vi "JTAG Test Panel.vi"() -> ()   [LabVIEW 2010]
uses:
  <vilib>/measure/NI_MABase.lvlib
  <vilib>/Analysis/NI_AALBase.lvlib
panel:
  out "ProgBar":dbl(slide) caption="Send to UUT..." scale=0.0..1.0
  in  "Tab Control":enum32{"General", "Stim"}(tab)=enum."Stim"
  in  "GoStorage":bool
  in  "DCO8MHz":bool
  in  "DCO1Mhz":bool
  in  "InitFirmware":bool
  in  "ResetFirmware":bool
  in  "InitJTAG":bool
  in  "ReadDefaults":bool
  in  "SetDefaults":bool
  out "Power ASIC Trim Values":string[][](table)=[["0x98"], ["0x14"], ["0xFF"], ["0x20"], ["0xFF"], ["0x20"], ["0x2D"], ["0x58"], ["0x1F"], ["0x00"], ["0x77"]]
  in  "BG_CTRL":bool
  in  "CG_CTRL":bool=TRUE
  in  "CG_CTRL 2":u8=170 format="%02x"
  in  "BG_CTRL 2":u8=128 format="%02x"
  in  "BC_CTRL1":u8=28 format="%02x"
  in  "BC_CTRL0":u8=20 max=64 step=1 format="%02x"
  in  "WFD_CTRL":u8=2 format="%02x"
  in  "Pulse Clock":bool
  in  "Pulses":u8=255
  in  "Stop Clock":bool
  in  "Calc Current":bool
  in  "CBAL 26":bool
  in  "UCS/S 26":bool
  in  "Enable 26":bool
  in  "Cal 26":bool
  in  "Current Ch 26":dbl format="%02_4f"
  in  "Direction 26":bool
  in  "Value Ch 26":u16 max=1023 step=1 format="%03x"
  in  "CBAL 25":bool
  in  "UCS/S 25":bool
  in  "Enable 25":bool
  in  "Cal 25":bool
  in  "Current Ch 25":dbl format="%02_4f"
  in  "Direction 25":bool
  in  "Value Ch 25":u16 max=1023 step=1 format="%03x"
  in  "CBAL 24":bool
  in  "UCS/S 24":bool
  in  "Enable 24":bool
  in  "Cal 24":bool
  in  "Current Ch 24":dbl format="%02_4f"
  in  "Direction 24":bool
  in  "Value Ch 24":u16 max=1023 step=1 format="%03x"
  in  "CBAL 23":bool
  in  "UCS/S 23":bool
  in  "Enable 23":bool
  in  "Cal 23":bool
  in  "Current Ch 23":dbl format="%02_4f"
  in  "Direction 23":bool
  in  "Value Ch 23":u16 max=1023 step=1 format="%03x"
  in  "CBAL 22":bool
  in  "UCS/S 22":bool
  in  "Enable 22":bool
  in  "Cal 22":bool
  in  "Current Ch 22":dbl format="%02_4f"
  in  "Direction 22":bool
  in  "Value Ch 22":u16 max=1023 step=1 format="%03x"
  in  "CBAL 21":bool
  in  "UCS/S 21":bool
  in  "Enable 21":bool
  in  "Cal 21":bool
  in  "Current Ch 21":dbl format="%02_4f"
  in  "Direction 21":bool
  in  "Value Ch 21":u16 max=1023 step=1 format="%03x"
  in  "CBAL 20":bool
  in  "UCS/S 20":bool
  in  "Enable 20":bool
  in  "Cal 20":bool
  in  "Current Ch 20":dbl format="%02_4f"
  in  "Direction 20":bool
  in  "Value Ch 20":u16 max=1023 step=1 format="%03x"
  in  "CBAL 19":bool
  in  "UCS/S 19":bool
  in  "Enable 19":bool
  in  "Cal 19":bool
  in  "Current Ch 19":dbl format="%02_4f"
  in  "Direction 19":bool
  in  "Value Ch 19":u16 max=1023 step=1 format="%03x"
  in  "CBAL 18":bool
  in  "UCS/S 18":bool
  in  "Enable 18":bool
  in  "Cal 18":bool
  in  "Current Ch 18":dbl format="%02_4f"
  in  "Direction 18":bool
  in  "Value Ch 18":u16 max=1023 step=1 format="%03x"
  in  "CBAL 17":bool
  in  "UCS/S 17":bool
  in  "Enable 17":bool
  in  "Cal 17":bool
  in  "Current Ch 17":dbl format="%02_4f"
  in  "Direction 17":bool
  in  "Value Ch 17":u16 max=1023 step=1 format="%03x"
  in  "CBAL 16":bool
  in  "UCS/S 16":bool
  in  "Enable 16":bool
  in  "Cal 16":bool
  in  "Current Ch 16":dbl format="%02_4f"
  in  "Direction 16":bool
  in  "Value Ch 16":u16 max=1023 step=1 format="%03x"
  in  "CBAL 15":bool
  in  "UCS/S 15":bool
  in  "Enable 15":bool
  in  "Cal 15":bool
  in  "Current Ch 15":dbl format="%02_4f"
  in  "Direction 15":bool
  in  "Value Ch 15":u16 max=1023 step=1 format="%03x"
  in  "CBAL 14":bool
  in  "UCS/S 14":bool
  in  "Enable 14":bool
  in  "Cal 14":bool
  in  "Current Ch 14":dbl format="%02_4f"
  in  "Direction 14":bool
  in  "Value Ch 14":u16 max=1023 step=1 format="%03x"
  in  "CBAL 13":bool
  in  "UCS/S 13":bool
  in  "Enable 13":bool
  in  "Cal 13":bool
  in  "Current Ch 13":dbl format="%02_4f"
  in  "Direction 13":bool
  in  "Value Ch 13":u16 max=1023 step=1 format="%03x"
  in  "CBAL 12":bool
  in  "UCS/S 12":bool
  in  "Enable 12":bool
  in  "Cal 12":bool
  in  "Current Ch 12":dbl format="%02_4f"
  in  "Direction 12":bool
  in  "Value Ch 12":u16 max=1023 step=1 format="%03x"
  in  "CBAL 11":bool
  in  "UCS/S 11":bool
  in  "Enable 11":bool
  in  "Cal 11":bool
  in  "Current Ch 11":dbl format="%02_4f"
  in  "Direction 11":bool
  in  "Value Ch 11":u16 max=1023 step=1 format="%03x"
  in  "CBAL 10":bool
  in  "UCS/S 10":bool
  in  "Enable 10":bool
  in  "Cal 10":bool
  in  "Current Ch 10":dbl format="%02_4f"
  in  "Direction 10":bool
  in  "Value Ch 10":u16 max=1023 step=1 format="%03x"
  in  "CBAL 9":bool
  in  "UCS/S 9":bool
  in  "Enable 9":bool
  in  "Cal 9":bool
  in  "Current Ch 9":dbl format="%02_4f"
  in  "Direction 9":bool
  in  "Value Ch 9":u16 max=1023 step=1 format="%03x"
  in  "CBAL 8":bool
  in  "UCS/S 8":bool
  in  "Enable 8":bool
  in  "Cal 8":bool
  in  "Current Ch 8":dbl format="%02_4f"
  in  "Direction 8":bool
  in  "Value Ch 8":u16 max=1023 step=1 format="%03x"
  in  "CBAL 7":bool
  in  "UCS/S 7":bool
  in  "Enable 7":bool
  in  "Cal 7":bool
  in  "Current Ch 7":dbl format="%02_4f"
  in  "Direction 7":bool
  in  "Value Ch 7":u16 max=1023 step=1 format="%03x"
  in  "CBAL 6":bool
  in  "UCS/S 6":bool
  in  "Enable 6":bool
  in  "Cal 6":bool
  in  "Current Ch 6":dbl format="%02_4f"
  in  "Direction 6":bool
  in  "Value Ch 6":u16 max=1023 step=1 format="%03x"
  in  "CBAL 5":bool
  in  "UCS/S 5":bool
  in  "Enable 5":bool
  in  "Cal 5":bool
  in  "Current Ch 5":dbl format="%02_4f"
  in  "Direction 5":bool
  in  "Value Ch 5":u16 max=1023 step=1 format="%03x"
  in  "CBAL 4":bool
  in  "UCS/S 4":bool
  in  "Enable 4":bool
  in  "Cal 4":bool
  in  "Current Ch 4":dbl format="%02_4f"
  in  "Direction 4":bool
  in  "Value Ch 4":u16 max=1023 step=1 format="%03x"
  in  "CBAL 3":bool
  in  "UCS/S 3":bool
  in  "Enable 3":bool
  in  "Cal 3":bool
  in  "Current Ch 3":dbl format="%02_4f"
  in  "Direction 3":bool
  in  "Value Ch 3":u16 max=1023 step=1 format="%03x"
  in  "CBAL 2":bool
  in  "UCS/S 2":bool
  in  "Enable 2":bool
  in  "Cal 2":bool
  in  "Current Ch 2":dbl format="%02_4f"
  in  "Direction 2":bool
  in  "Value Ch 2":u16 max=1023 step=1 format="%03x"
  in  "CBAL 1":bool
  in  "UCS/S 1":bool
  in  "Enable 1":bool
  in  "Cal 1":bool
  in  "Current Ch 1":dbl format="%02_4f"
  in  "Direction 1":bool
  in  "Value Ch 1":u16 max=1023 step=1 format="%03x"
  in  "RST":bool=TRUE
  in  "SEL":bool
  in  "CONT":bool
  in  "STOP":bool
  in  "RUN":bool
  in  "Status Polling":bool=TRUE
  out "ACTIVE":bool
  out "ERR_N":bool
  out "PAUSE":bool
  out "SYNC":bool
  out "PROG":bool
  out "WPF":bool
  out "RVF":bool
  out "ADRF":bool
  out "SEQF":bool
  out "PARF":bool
  out "PGF":bool
  in  "RAM2 Peak":u8=255 format="%x"
  in  "Set RAM 2":bool
  in  "RAM 2 SHAPE":u16(ring) items=["Zero", "Full", "Sine", "Haversine", "Triangle", "Pos Ramp", "Neg Ramp", "Noise", "Sine Sweep"]
  out "SEQ2 Waveform":dbl[](graph)
  in  "RAM1 Peak":u8=255 format="%x"
  in  "Set RAM 1":bool
  in  "RAM 1 SHAPE":u16(ring) items=["Zero", "Full", "Sine", "Haversine", "Triangle", "Pos Ramp", "Neg Ramp", "Noise", "Sine Sweep"]
  out "SEQ1 Waveform":dbl[](graph)
  in  "Shutdown UUT":bool
  in  "High Voltage is:":bool=TRUE
  in  "PG (n*128uS, 0=OFF)":u8 max=127 step=1 format="%02x"
  in  "Clock Divider Enabled:":bool=TRUE
  in  "Clock Divisor(n+1):":u8 max=127 step=1 format="%02x"
  in  "Phase Offset:":u8 step=1 format="%02x"
  in  "STPC":u8=1 step=1 format="%02x"
  in  "STPB+STPA":u16 step=1 format="%04x"
  in  "PAUSE after PHASE:":bool
  in  "SYNC Sends:":bool
  in  "Phase Repetitions:":u8(ring) items=["1", "2", "3", "4", "5", "6", "7", "8", "9", "10", "11", "12", "13", "14", "15", "16"]
  in  "Delay/Pause Flag:":bool
  in  "Uncontrolled":bool
  in  "WFM Source:":u8(ring) items=["Rectangle 1", "Rectangle 2", "Rectangle 3", "Rectangle 4", "Rectangle 5", "Rectangle 6", "RAM 1", "RAM 2"]
  in  "PHASE":u8=1 min=1 max=24 step=1
  in  "Trailing Delay(n+1CLK):":u16 step=1 format="%04x"
  in  "Set Basic Enables":bool=TRUE
  in  "Set All RVLD Bits":bool=TRUE
  in  "Ph/Seq/Ram Wr Ena":bool=TRUE
  in  "Set PGOE Bit":bool=TRUE
  in  "Set WGE Bit":bool=TRUE
  in  "Starting Phase 1":u8(ring)=7 items=["1", "2", "3", "4", "5", "6", "7", "8", "9", "10", "11", "12", "13", "14", "15", "16", "17", "18", "19", "20", "21", "22", "23", "24"]
  in  "Ending Phase 1":u8(ring)=8 items=["1", "2", "3", "4", "5", "6", "7", "8", "9", "10", "11", "12", "13", "14", "15", "16", "17", "18", "19", "20", "21", "22", "23", "24"]
  in  "Ending Phase 0":u8(ring)=1 items=["1", "2", "3", "4", "5", "6", "7", "8", "9", "10", "11", "12", "13", "14", "15", "16", "17", "18", "19", "20", "21", "22", "23", "24"]
  in  "Starting Phase 0":u8(ring) items=["1", "2", "3", "4", "5", "6", "7", "8", "9", "10", "11", "12", "13", "14", "15", "16", "17", "18", "19", "20", "21", "22", "23", "24"]
  in  "Clear":bool
  in  "Download":bool
  in  "Reset":bool
  in  "Load":bool
  in  "Save":bool
  in  "RECT 6":u8=255 max=127 step=1 format="%02x"
  in  "RECT 5":u8=255 max=127 step=1 format="%02x"
  in  "RECT 4":u8=255 max=127 step=1 format="%02x"
  in  "RECT 3":u8=255 max=127 step=1 format="%02x"
  in  "RECT 2":u8=255 max=127 step=1 format="%02x"
  in  "RECT 1":u8=255 max=127 step=1 format="%02x"
  out "ProgBar 2":dbl(slide) caption="Send to UUT..." scale=0.0..1.0
  out "error out":errorcluster
  in  "error in (no error)":errorcluster
  # "UNCONTR\nSRC/SINK"
  # "ENABLED"
  # "CHG BAL"
  # "Channel Output Assignments For This Phase"
  # "DIR"
  # "AMPL"
  # "CAL"
  # "mA"
  # "mA"
  # "mA"
  # "mA"
  # "mA"
  # "Saturn Phase Programmer"
  # "mA"
  # "mA"
  # "mA"
  # "mA"
  # "mA"
  # "mA"
  # "mA"
  # "mA"
  # "mA"
  # "mA"
  # "mA"
  # "mA"
  # "mA"
  # "mA"
  # "mA"
  # "mA"
  # "mA"
  # "mA"
  # "mA"
  # "mA"
  # "mA"
  # "Power Registers"
  # "H"
  # "L"
  # "H"
  # "L"
  # "H"
  # "L"
  # "H"
  # "L"
  # "H"
  # "L"
  # "."
  # "Phase Step Size:"
  # "Enables"
  # "Program Sequence"
  # "Rectangle\nAmplitudes"
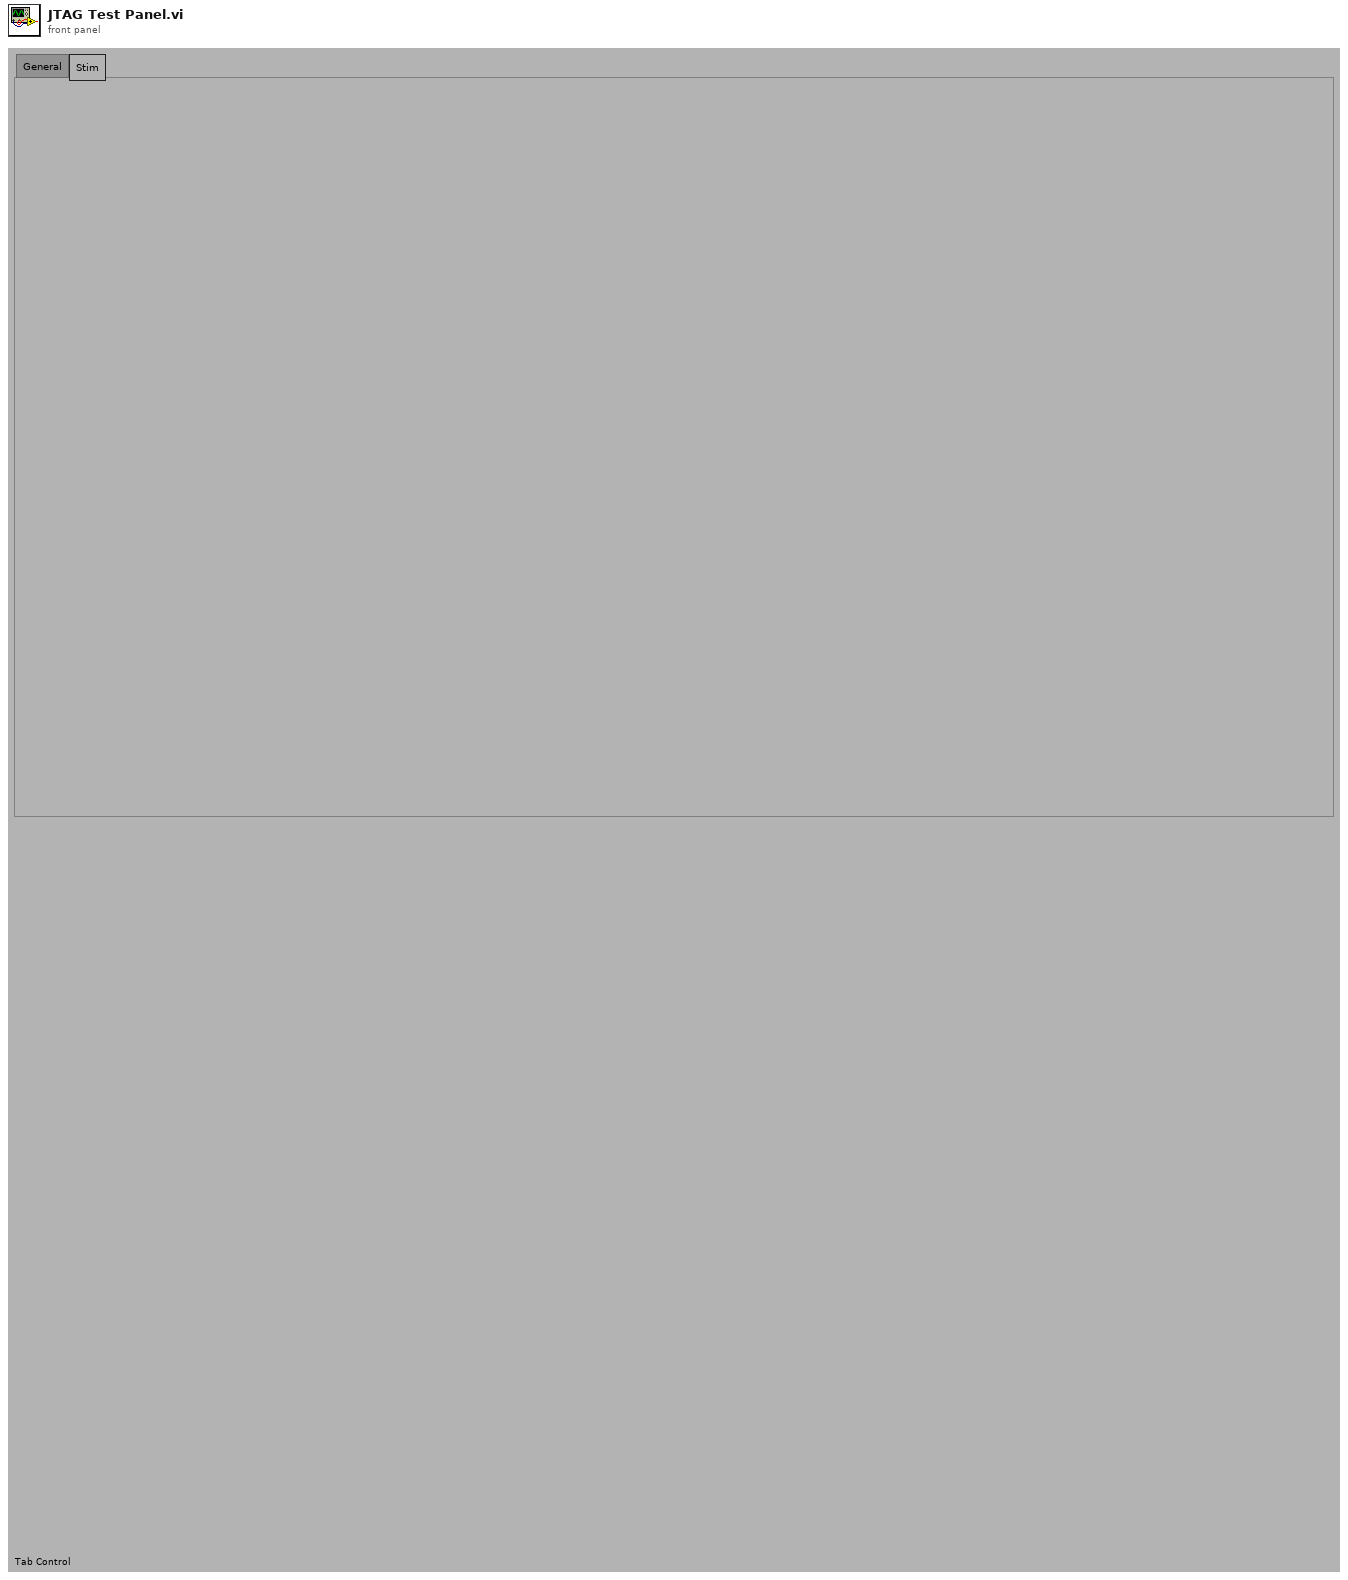
[diagram p1: front panel]
types:
  T1 = cluster{"PHASE Changed":bool, "BASE Changed":bool, "SEQ Changed":bool, "PHASE":u8, "STOP":bool, "RUN":bool, "CONT":bool, "SEL":bool, "Stop Clock":bool, "Output Caps Shorted:":bool, "Override Changes":bool, "UUT is UP":bool, "Channel Loads:":bool, "Downlink Progress":i32, "RAM 1 SHAPE":u16, "RAM 2 SHAPE":u16, "RAM1":u8[], "RAM2":u8[], "RST":bool, "Pulse":bool}
  T2 = enum16{"Sine Wave", "Triangle Wave", "Square Wave", "Sawtooth Wave"}
  T3 = cluster{"frequency":dbl, "amplitude":dbl, "phase":dbl}[]
  T4 = enum8{"PORT_OUT", "PORT_SEL", "PORT_RES_EN", "READ_PORT", "PORT_DIR", "SET_LCM", "PLUTO_WRITE_SINGLE", "PLUTO_READ_SINGLE", "PLUTO_WRITE_MASK", "STIM_POWER_UP", "STIM_POWER_DN", "SATURN_WRITE_SINGLE", "SATURN_READ_SINGLE", "SATURN_WRITE_BLOCK", "SATURN_READ_BLOCK", "SATURN_WRITE_MASK", "MICS_POWER_UP", "MICS_POWER_DN", "MICS_WRITE_SINGLE", "MICS_READ_SINGLE", "MICS_WRITE_BLOCK", "MICS_READ_BLOCK", "MICS_WRITE_MASK", "MEM_POWER_UP", "MEM_POWER_DN", "MEM_WRITE_SINGLE", "MEM_READ_SINGLE", "MEM_WRITE_BLOCK", "MEM_READ_BLOCK", "MEM_WRITE_MASK", "MEM_WRITE_SR", "MEM_READ_SR", "MEM_OPCODE", "INIT_VARIABLES", "DCO -> 1 MHz", "DCO -> 8 MHz", "START_STIM_CLK", "STOP_STIM_CLK", "PULSE_STIM_CLK", "PULSE_STIM_SCK", "SINGLE_ADC12", "SINGLE_ADC12_REPEAT", "MULTI_ADC12", "MULTI_ADC12_REPEAT", "Disable_ADC12", "READ_IO_VARIABLES"}
  T5 = enum8{"Port 1", "Port 2", "Port 3", "Port 4", "Port 5", "Port 6", "Port 7", "Port 8"}
  T6 = enum16{"Manual Inputs", "PWR_LDO_EN", "PWR_STROBE_IN", "PWR_UV_PROT", "PWR_MAG_TO_OVRD", "PWR_BBC_CTL", "PWR_HVDD_CONN", "<Reserved_1>", "<Reserved_2>", "STIM_RUN", "STIM_STOP", "STIM_CONT", "STIM_SEL", "RST_N", "<Reserved_3>", "TETS_TXD", "<Reserved_4>", "<Reserved_5>", "PWR_MAG_SW (IN)", "PWR_MAG_2S (IN)", "PWR_MAG_5S (IN)", "TETS_RXD (IN)", "PWR_V_DET (IN)", "PWR_BRWN_OUT (IN)", "MICS_IRQ", "<Reserved_7>", "STIM_PROG (IN)", "STIM_PAUSE (IN)", "STIM_SYNC (IN)", "STIM_TFLG (IN)", "STIM_ERR (IN)"}
  T7 = enum16{"PWR LDOA_EN BIT", "PWR VD1_EN BIT", "PWR VD2_EN BIT", "PWR VD3_EN BIT", "PWR VD4_EN BIT", "PWR BFG_EN BIT", "PWR TEMP_EN BIT", "PWR THERM_EN BIT", "PWR CHARGE_EN BIT", "PWR COMP_OV BIT", "PWR MSPBUF < MSPBUF_IN", "PWR MSPBUF < Fuel Gauge", "PWR MSPBUF < Recharge PM", "PWR MSPBUF < Temp_Out", "PWR MSPBUF < Therm_Bias", "PWR MSPBUF < Therm_Input", "PWR MSPBUF < Therm_Offset", "PWR MSPBUF OFF", "PWR ASK_POL BIT", "PWR MAGSW_DISABLE BIT", "PWR MAGTIME_SEL 00 (OFF)", "PWR MAGTIME_SEL 01 (5S)", "PWR MAGTIME_SEL 10 (2S)", "PWR MAGTIME_SEL 11 (TEST)", "PWR STROBE_INT_EN BIT", "PWR STROBE_PW SET", "PWR STROBE_FREQ SET", "PWR HCM_PW SET", "PWR LCM_DC SET"}
  T8 = cluster{"Enable":bool[], "UCS/S":bool[], "CBAL":bool[], "Direction":bool[], "Value":u16[], "CAL":bool[], "Waveform Source:":u8, "Phase Repetitions:":u8, "SYNC Sends:":bool, "Delay/Pause Flag:":bool, "Uncontrolled":bool, "Clock Divider Enabled:":bool, "Clock Divisor(n+1):":u8, "STPC":u8, "STPB+STPA":u16, "PAUSE after PHASE:":bool, "Trailing Delay(n+1CLK):":u16, "Pulse Guard (n*128uS, 0=OFF)":u8, "Phase Offset:":u8, "High Voltage is:":bool}
  T9 = enum16{"Read Port Value", "Set Port Value", "Set Port Direction", "Set Port Select", "Set Port Res En"}
  T10 = cluster{"Enable":bool[], "UCS/S":bool[], "CBAL":bool[], "Direction":bool[], "Value":u16[], "CAL":bool[], "Waveform Source:":u8, "Phase Repetitions:":u8, "SYNC Sends:":bool, "Delay/Pause Flag:":bool, "Uncontrolled":bool, "Clock Divider Enabled:":bool, "Clock Divisor(n+1):":u8, "STPC":u8, "STPB+STPA":u16, "PAUSE after PHASE:":bool, "Trailing Delay(n+1CLK):":u16, "Pulse Guard (n*128uS, 0=OFF)":u8, "Phase Offset:":u8, "High Voltage is:":bool}[]
  T11 = cluster{"Set RAM 1":bool, "Set RAM 2":bool, "RAM 1 SHAPE":u16, "RAM 2 SHAPE":u16, "RECT 1":u8, "RECT 2":u8, "RECT 3":u8, "RECT 4":u8, "RECT 5":u8, "RECT 6":u8, "WaveDAC Ref Current":u8, "Set Basic Enables":bool, "Ph/Seq/Ram Wr Ena":bool, "Set WGE Bit":bool, "Set All RVLD Bits":bool, "Set PGOE Bit":bool, "Starting Phase 0":u8, "Ending Phase 0":u8, "Starting Phase 1":u8, "Ending Phase 1":u8, cluster{"Enable":bool[], "UCS/S":bool[], "CBAL":bool[], "Direction":bool[], "Value":u16[], "CAL":bool[], "Waveform Source:":u8, "Phase Repetitions:":u8, "SYNC Sends:":bool, "Delay/Pause Flag:":bool, "Uncontrolled":bool, "Clock Divider Enabled:":bool, "Clock Divisor(n+1):":u8, "STPC":u8, "STPB+STPA":u16, "PAUSE after PHASE:":bool, "Trailing Delay(n+1CLK):":u16, "Pulse Guard (n*128uS, 0=OFF)":u8, "Phase Offset:":u8, "High Voltage is:":bool}[], "Addresses":u16[], "Data":u8[]}
  T12 = cluster{"RECT 1":u8, "RECT 2":u8, "RECT 3":u8, "RECT 4":u8, "RECT 5":u8, "RECT 6":u8, "WaveDAC Ref Current":u8, "Set Basic Enables":bool, "Ph/Seq/Ram Wr Ena":bool, "Set WGE Bit":bool, "Set All RVLD Bits":bool, "Set PGOE Bit":bool, "Starting Phase 0":u8, "Ending Phase 0":u8, "Starting Phase 1":u8, "Ending Phase 1":u8}
  T13 = cluster{"Set RAM 1":bool, "Set RAM 2":bool, "RAM 1 SHAPE":u16, "RAM 2 SHAPE":u16}
  T14 = enum8{"Enabled", "Disabled", "Disabled and Grayed Out"}
  T15 = cluster{"Boolean array[0]":bool, "Boolean array[1]":bool, "Boolean array[2]":bool, "Boolean array[3]":bool, "Boolean array[4]":bool, "Boolean array[5]":bool, "Boolean array[6]":bool, "Boolean array[7]":bool, "Boolean array[8]":bool}
  T16 = cluster{"RECT 1":u8, "RECT 2":u8, "RECT 3":u8, "RECT 4":u8, "RECT 5":u8, "RECT 6":u8, "WFD_CTRL":u8, "Set Basic Enables":bool, "Ph/Seq/Ram Wr Ena":bool, "Set WGE Bit":bool, "Set All RVLD Bits":bool, "Set PGOE Bit":bool, "Starting Phase 0":u8, "Ending Phase 0":u8, "Starting Phase 1":u8, "Ending Phase 1":u8}
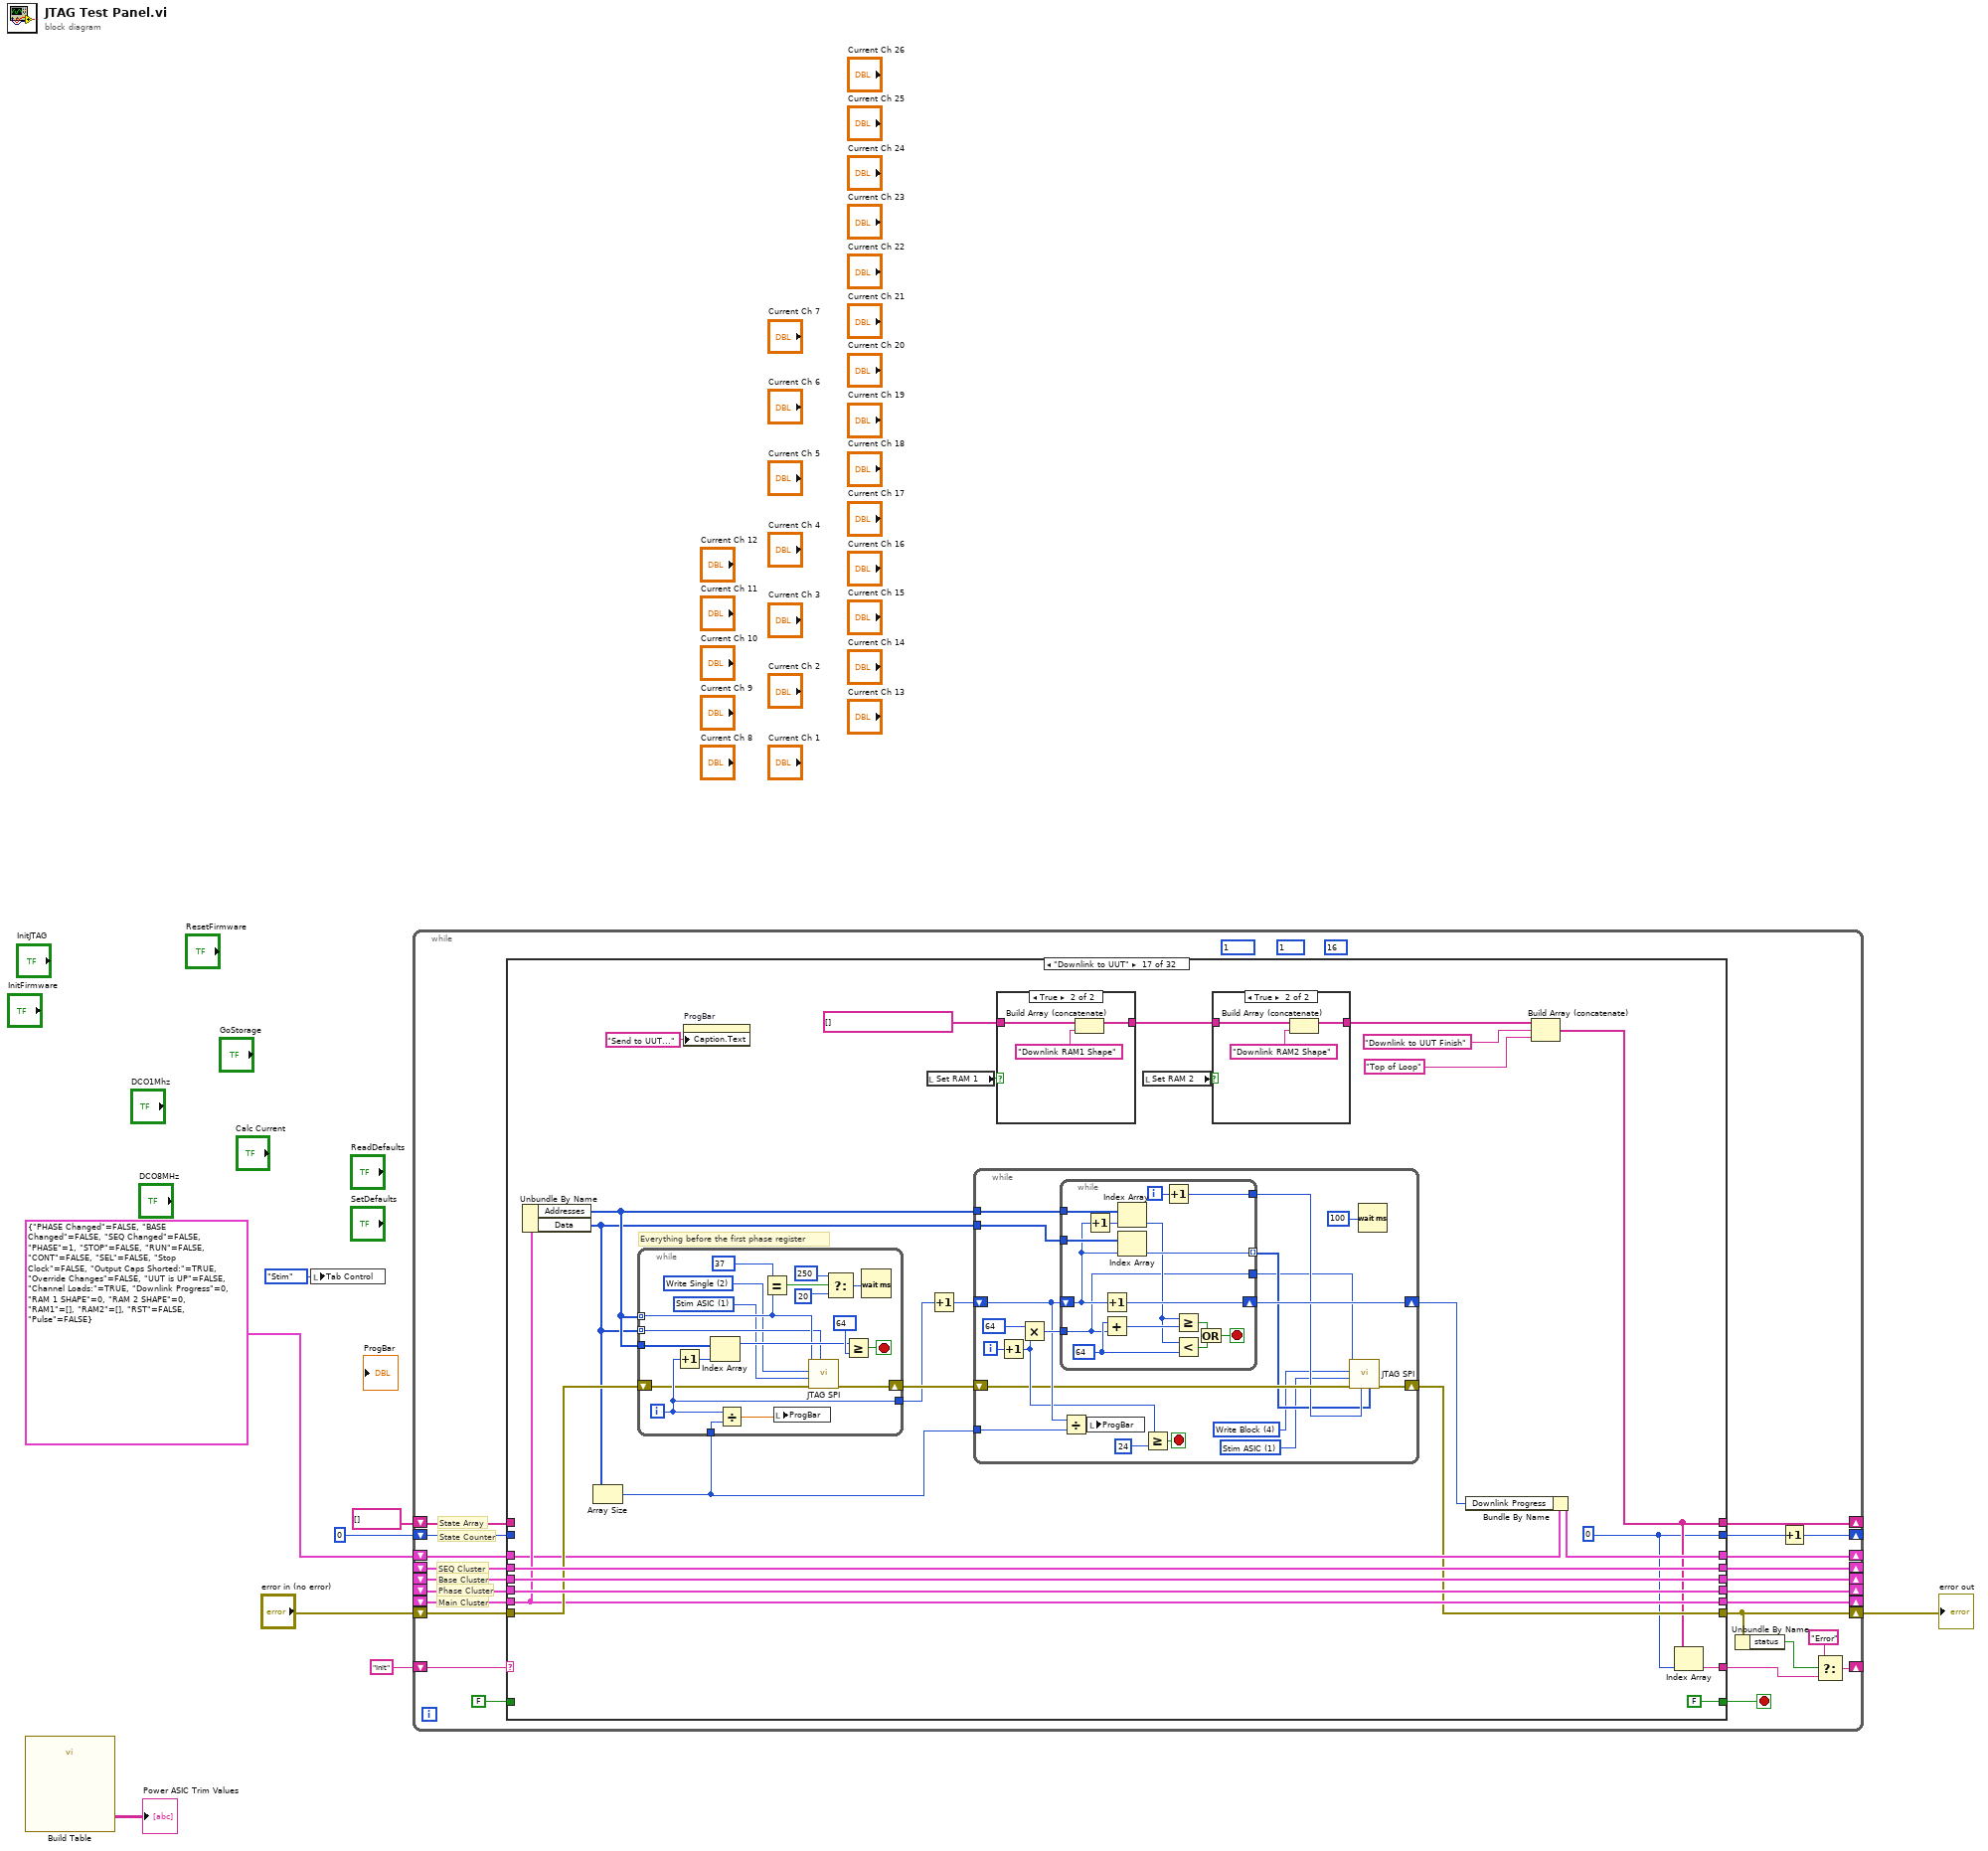
[diagram p0: block diagram]
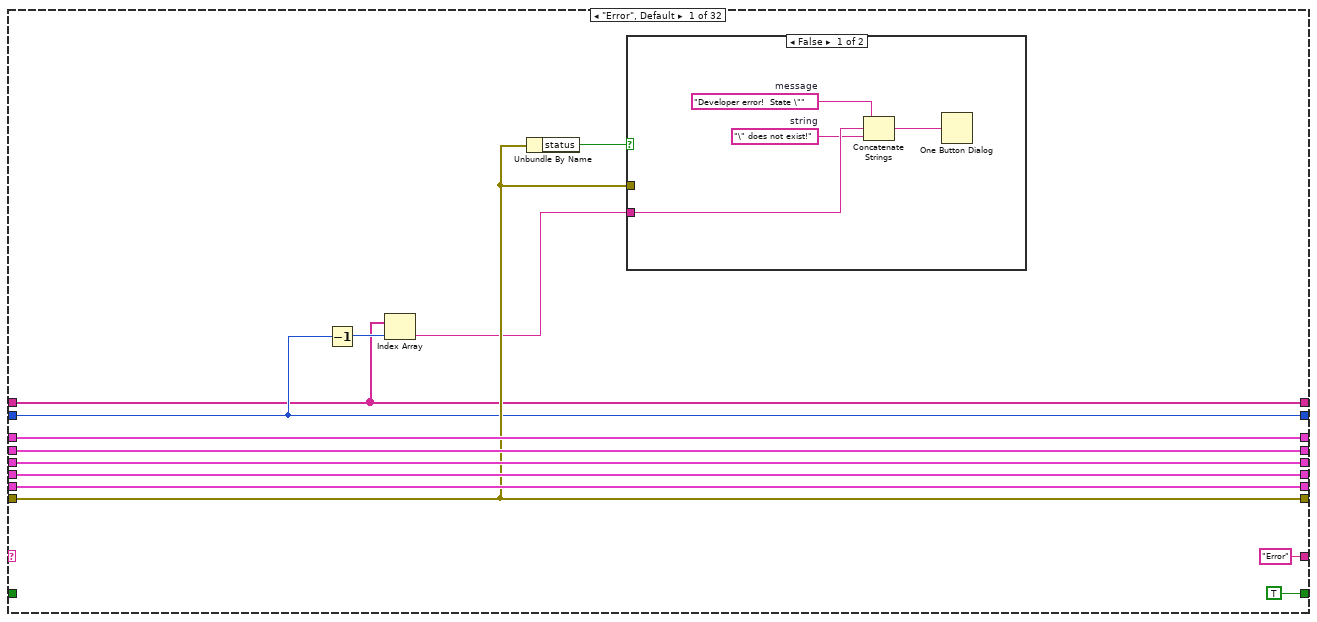
[diagram p2: hidden frame]
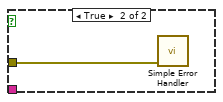
[diagram p3: hidden frame]
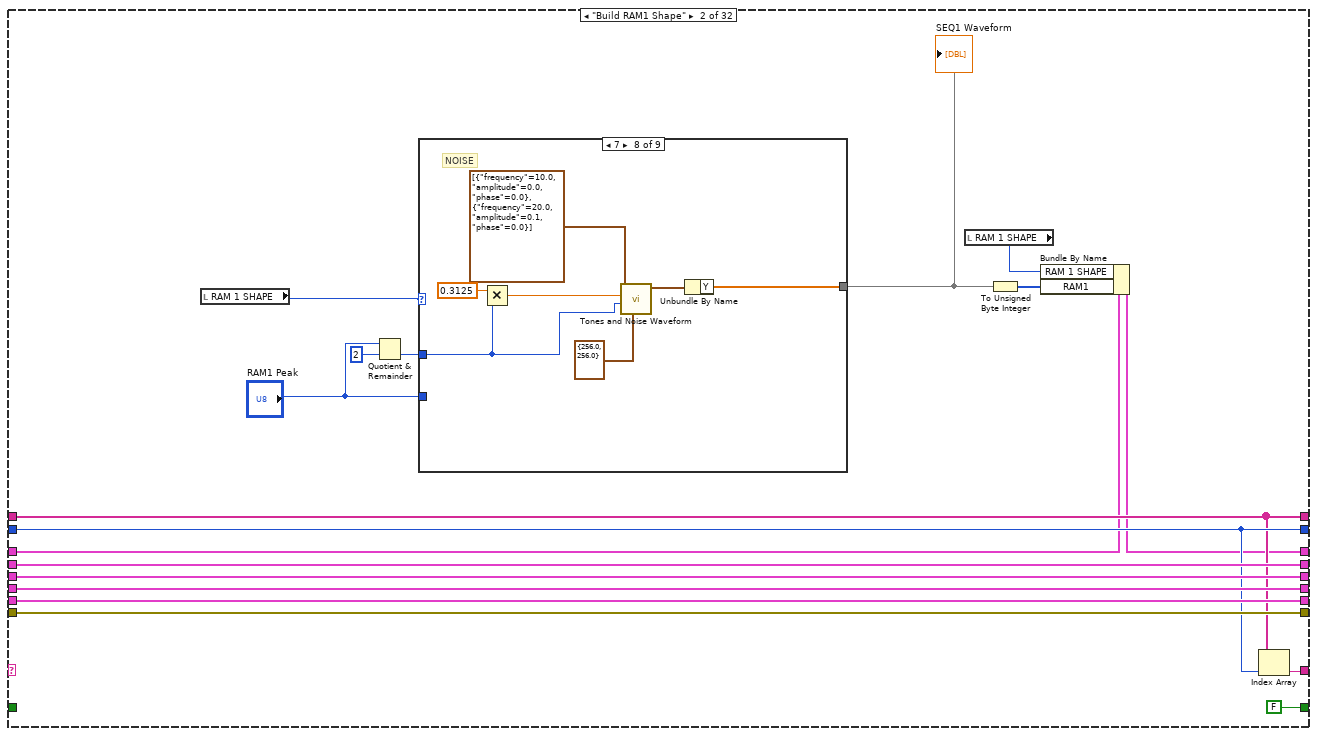
[diagram p4: hidden frame]
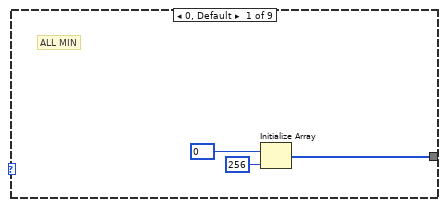
[diagram p5: hidden frame]
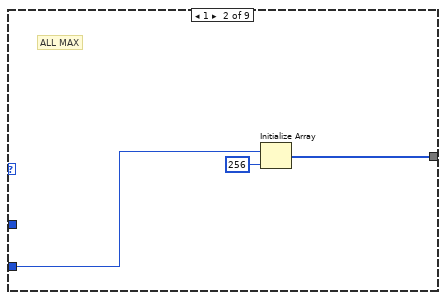
[diagram p6: hidden frame]
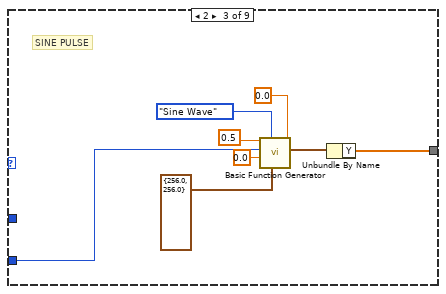
[diagram p7: hidden frame]
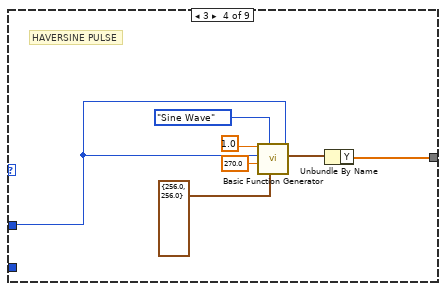
[diagram p8: hidden frame]
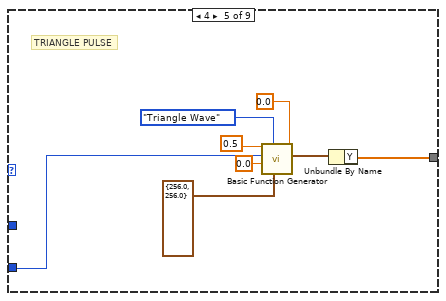
[diagram p9: hidden frame]
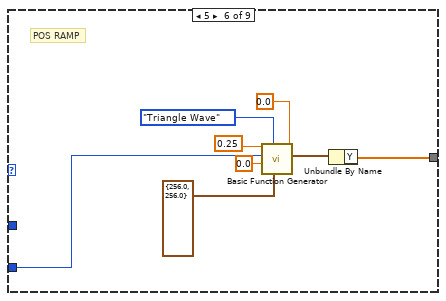
[diagram p10: hidden frame]
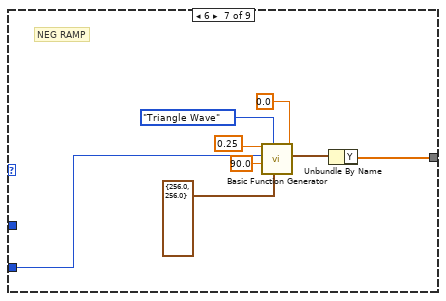
[diagram p11: hidden frame]
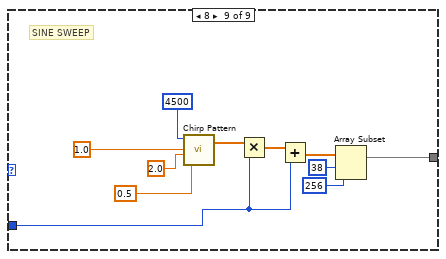
[diagram p12: hidden frame]
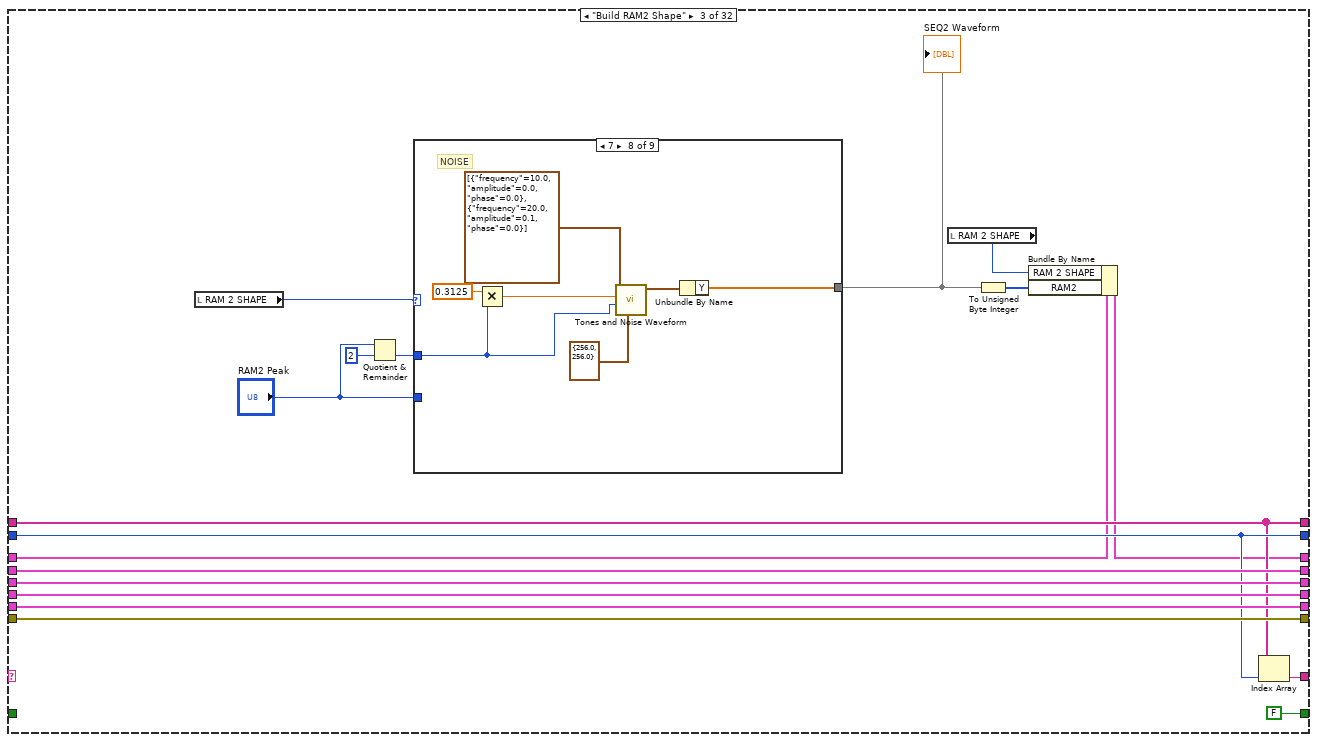
[diagram p13: hidden frame]
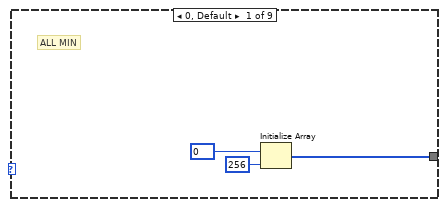
[diagram p14: hidden frame]
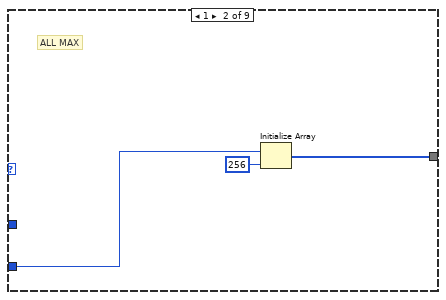
[diagram p15: hidden frame]
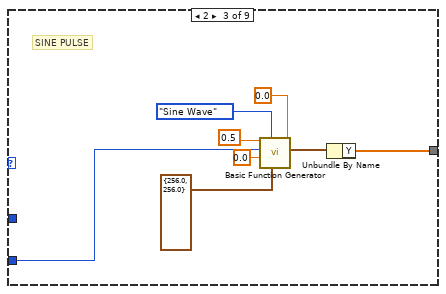
[diagram p16: hidden frame]
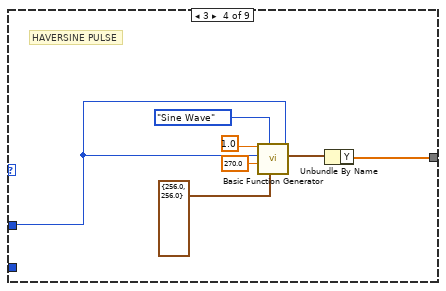
[diagram p17: hidden frame]
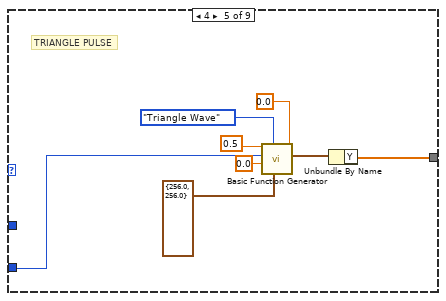
[diagram p18: hidden frame]
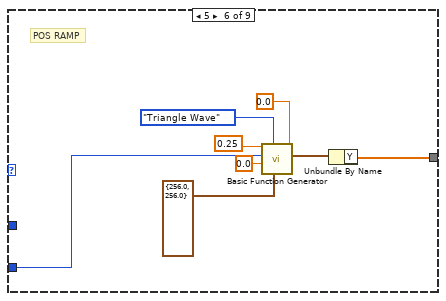
[diagram p19: hidden frame]
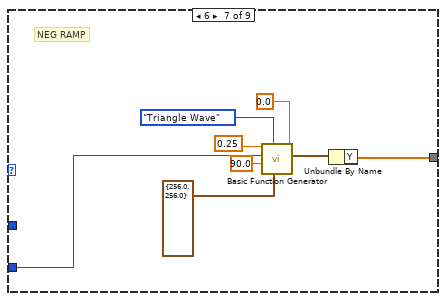
[diagram p20: hidden frame]
diagram:
  n1 = call "Build Table"() -> ("Table"=→"Power ASIC Trim Values":string[][])  [unwired: 10 in, 1 out]
  n2 = local write "Tab Control"(enum32{"General", "Stim"}."Stim" ("Tab Control")) -> ()
  n3 = while {
    shift-right: [w28] -> _
    shift-left: _ -> [w32]
    shift-right: [w27] -> _
    shift-left: _ -> [w31]
    shift-right: [w26] -> _
    shift-left: _ -> [w30]
    shift-right: [w20] -> w6
    shift-left: "error in (no error)" -> [w29]
    shift-right: [w22] -> _
    shift-left: "Init" -> [w25]
    shift-right: [w16] -> _
    shift-left: _ -> [w17]
    shift-right: [w14] -> _
    shift-left: T1 {"PHASE Changed"=FALSE, "BASE Changed"=FALSE, "SEQ Changed"=FALSE, "PHASE"=1, "STOP"=FALSE, "RUN"=FALSE, "CONT"=FALSE, "SEL"=FALSE, "Stop Clock"=FALSE, "Output Caps Shorted:"=TRUE, "Override Changes"=FALSE, "UUT is UP"=FALSE, "Channel Loads:"=TRUE, "Downlink Progress"=0, "RAM 1 SHAPE"=0, "RAM 2 SHAPE"=0, "RAM1"=[], "RAM2"=[], "RST"=FALSE, "Pulse"=FALSE} -> [w15]
    shift-right: [w10] -> _
    shift-left: u8 0 -> [w13]
    shift-right: [w9] -> _
    shift-left: string[] [] -> [w12]
    stop <- w24 stop-if-true
    (unwired) u8 16
    (unwired) u16 1 ("SPI Address")
    (unwired) u16 1 ("SPI Address")
    # "State Counter"
    # "State Array"
    # "SEQ Cluster"
    # "Base Cluster"
    # "Phase Cluster"
    # "Main Cluster"
    n4 = case shown="\"Downlink to UUT\"" w25 {
      tunnel: w32 -> [w45 w68 w149 w225 w259 w297 w324 w353 w367 w375 w416 w428 w440 w452 w464 w491 w518 w597 w633 w1143 w1178 w1226 w1266 w1449 _ w1500 w1517 w1557 _ w1783 w1962 w1980]
      tunnel: w31 -> [w44 w67 w148 w224 w258 w296 w323 w352 w366 w376 w415 w427 w439 w451 w463 w490 w517 w596 w632 w1142 _ _ w1265 w1423 w1479 w1505 w1516 w1551 _ w1757 w1961 w1979]
      tunnel: w30 -> [w43 w66 w147 w223 w257 w290 w322 w351 w365 w372 w414 w426 w438 w450 w462 w489 w512 w595 w603 w1126 w1153 w1215 w1264 _ w1470 w1504 w1515 w1521 w1748 w1784 w1960 w1968]
      tunnel: w29 -> [w37 w63 w144 w214 w249 w284 w318 w342 w356 w371 w406 w417 w429 w441 w453 w479 w513 w585 w631 w1125 w1154 w1225 w1245 w1452 w1478 w1503 w1506 w1556 w1755 w1785 w1959 w1978]
      tunnel: [w45 w68 w149 w225 w259 w297 w324 w353 w367 w375 w416 w428 w440 w452 w464 w491 w518 w597 w633 w1143 w1177 w1226 w1266 w1449 w1475 w1500 w1517 w1557 w1737 w1783 w1962 w1980] -> w28
      tunnel: [w44 w67 w148 w224 w258 w296 w323 w352 w366 w376 w415 w427 w439 w451 w463 w490 w517 w596 w632 w1142 w1181 w1221 w1265 w1423 w1479 w1505 w1516 w1523 w1743 w1757 w1961 w1979] -> w27
      tunnel: [w43 w66 w147 w223 w257 w290 w322 w351 w365 w372 w414 w426 w438 w450 w462 w489 w512 w595 w602 w1126 w1152 w1215 w1264 w1425 w1469 w1504 w1515 w1520 w1747 w1784 w1960 w1967] -> w26
      tunnel: [w37 w63 w144 w213 w247 w283 w318 w341 w355 w370 w381 w417 w429 w441 w453 w476 w501 w586 w631 w1127 w1188 w1225 w1245 w1452 w1478 w1503 w1506 w1556 w1755 w1785 w1959 w1978] -> w20
      tunnel: [TRUE FALSE FALSE FALSE FALSE FALSE FALSE FALSE FALSE w380 FALSE FALSE FALSE FALSE FALSE FALSE FALSE FALSE FALSE FALSE FALSE FALSE w1255 FALSE w1474 w1483 w1514 w1555 FALSE w1778 w1958 w1977] -> w24
      tunnel: FALSE -> [_ _ _ _ _ _ _ _ _ w380 _ _ _ _ _ _ _ _ _ _ _ _ w1255 _ w1474 w1483 w1514 w1555 _ w1778 w1958 w1977]
      tunnel: ["Error" w62 w143 w220 w254 w293 w317 w348 w362 w379 w411 w423 w435 w447 w459 w486 w514 w592 w627 w1138 w1199 w1218 w1256 w1414 w1473 w1482 w1507 w1529 w1752 w1781 w1952 w1976] -> w21
      tunnel: w17 -> [w42 w65 w146 w222 w256 w295 w321 w350 w364 w374 w413 w425 w437 w449 w461 w488 w516 w594 w630 w1141 w1160 w1224 w1263 w1450 w1477 w1502 w1513 w1554 _ w1782 w1957 w1972]
      tunnel: [w42 w65 w146 w222 w256 w295 w321 w350 w364 w374 w413 w425 w437 w449 w461 w488 w516 w594 w630 w1141 w1159 w1224 w1263 w1450 w1477 w1502 w1513 w1554 w1742 w1782 w1957 w1973] -> w16
      tunnel: w15 -> [w40 w59 w139 w217 w251 w286 w320 w345 w359 w373 w408 w420 w432 w444 w456 w483 w504 w589 w629 w1140 w1184 w1220 w1239 w1422 w1476 w1501 w1512 w1522 w1754 w1777 w1949 w1971]
      tunnel: [w40 w58 w138 w217 w251 w286 w320 w344 w358 w373 w407 w419 w431 w443 w455 w482 w503 w588 w629 w1140 w1187 w1219 w1242 w1421 w1476 w1501 w1511 w1550 w1754 w1777 w1949 w1970] -> w14
      tunnel: w13 -> [w36 w61 w142 w219 w253 w292 _ w346 w360 w377 w409 w421 w433 w445 w457 w484 _ w590 w625 w1136 w1197 w1216 _ w1413 w1471 w1480 _ w1527 w1750 w1779 w1950 w1974]
      tunnel: w12 -> [w34 w60 w141 w218 w252 w291 _ w347 w361 w378 w410 w422 w434 w446 w458 w485 _ w591 w626 w1137 w1198 w1217 _ w1412 w1472 w1481 _ w1528 w1751 w1780 w1951 w1975]
      tunnel: [w36 w61 w142 w219 w253 w292 w313 w346 w360 w377 w409 w421 w433 w445 w457 w484 w492 w590 w625 w1136 w1197 w1216 w1257 w1413 w1471 w1480 w1508 w1527 w1750 w1779 w1950 w1974] -> w11
      tunnel: [w34 w60 w141 w218 w252 w291 w314 w347 w361 w378 w410 w422 w434 w446 w458 w485 w493 w591 w626 w1137 w1198 w1217 w1258 w1412 w1472 w1481 w1509 w1528 w1751 w1780 w1951 w1975] -> w9
      frame "Error", Default {
        n5 = Decrement(x=w36) -> (x-1=w35:i32)
        n6 = Index Array(array=w34, index=w35) -> (element=w33:string)
        n7 = Unbundle By Name(w37) -> ("status"=w38:bool)
        n8 = case shown="False" w38 {
          tunnel: w37 -> [_ w50]
          tunnel: w33 -> [w48 _]
          frame False {
            w47 = "\" does not exist!"  # string
            w49 = "Developer error!  State \""  # message
            n9 = Concatenate Strings(w49, w48, w47) -> (w46:string)
            n10 = One Button Dialog(message=w46) -> ()  [unwired: 1 in, 1 out]
          }
          frame True {
            n11 = call <vilib>:"Simple Error Handler.vi"("error in (no error)"=w50) -> ()  [unwired: 4 in, 5 out]
          }
        }
      }
      frame "Build RAM1 Shape" {
        n12 = local read "RAM 1 SHAPE"() -> (w52:u16)
        n13 = Quotient & Remainder(x="RAM1 Peak", y=u8 2) -> (floor(x/y)=w55:u8)  [unwired: 1 out]
        n14 = case shown="7" w52 {
          tunnel: [w69 w73 w76 w84 w91 w99 w107 w118 w122] -> w51
          tunnel: "RAM1 Peak" -> [_ w72 w75 _ w90 w98 w106 _ _]
          tunnel: w55 -> [_ _ _ w83 _ _ _ w116 w121]
          frame 0, Default {
            # "ALL MIN"
            n15 = Initialize Array(u8 0, 256 ("dimension size")) -> (w69:u8[])
          }
          frame 1 {
            # "ALL MAX"
            n16 = Initialize Array(w72, 256 ("dimension size")) -> (w73:u8[])
          }
          frame 2 {
            # "SINE PULSE"
            n17 = call <vilib>:"Basic Function Generator.vi"("offset"=0.0, "sampling info"=cluster{"Fs":dbl, "#s":dbl} {"Fs"=256.0, "#s"=256.0}, "signal type"=T2."Sine Wave", "phase"=0.0, "amplitude"=w75, "frequency"=0.5) -> ("signal out"=w77:waveform(dbl))  [unwired: 3 in, 2 out]
            n18 = Unbundle By Name(w77) -> ("Y"=w76:dbl[])
          }
          frame 3 {
            # "HAVERSINE PULSE"
            n19 = call <vilib>:"Basic Function Generator.vi"("offset"=w83, "sampling info"=cluster{"Fs":dbl, "#s":dbl} {"Fs"=256.0, "#s"=256.0}, "signal type"=T2."Sine Wave", "phase"=270.0, "amplitude"=w83, "frequency"=1.0) -> ("signal out"=w85:waveform(dbl))  [unwired: 3 in, 2 out]
            n20 = Unbundle By Name(w85) -> ("Y"=w84:dbl[])
          }
          frame 4 {
            # "TRIANGLE PULSE"
            n21 = call <vilib>:"Basic Function Generator.vi"("offset"=0.0, "sampling info"=cluster{"Fs":dbl, "#s":dbl} {"Fs"=256.0, "#s"=256.0}, "signal type"=T2."Triangle Wave", "phase"=0.0, "amplitude"=w90, "frequency"=0.5) -> ("signal out"=w92:waveform(dbl))  [unwired: 3 in, 2 out]
            n22 = Unbundle By Name(w92) -> ("Y"=w91:dbl[])
          }
          frame 5 {
            # "POS RAMP"
            n23 = call <vilib>:"Basic Function Generator.vi"("offset"=0.0, "sampling info"=cluster{"Fs":dbl, "#s":dbl} {"Fs"=256.0, "#s"=256.0}, "signal type"=T2."Triangle Wave", "phase"=0.0, "amplitude"=w98, "frequency"=0.25) -> ("signal out"=w100:waveform(dbl))  [unwired: 3 in, 2 out]
            n24 = Unbundle By Name(w100) -> ("Y"=w99:dbl[])
          }
          frame 6 {
            # "NEG RAMP"
            n25 = call <vilib>:"Basic Function Generator.vi"("offset"=0.0, "sampling info"=cluster{"Fs":dbl, "#s":dbl} {"Fs"=256.0, "#s"=256.0}, "signal type"=T2."Triangle Wave", "phase"=90.0, "amplitude"=w106, "frequency"=0.25) -> ("signal out"=w108:waveform(dbl))  [unwired: 3 in, 2 out]
            n26 = Unbundle By Name(w108) -> ("Y"=w107:dbl[])
          }
          frame 7 {
            # "NOISE"
            n27 = Multiply(x=0.3125, y=w116) -> (x*y=w115:dbl)
            n28 = call <vilib>:"Tones and Noise Waveform.vi"("sampling info"=cluster{"Fs":dbl, "#s":dbl} {"Fs"=256.0, "#s"=256.0}, "offset"=w116, "noise (rms)"=w115, "tones"=T3 [{"frequency"=10.0, "amplitude"=0.0, "phase"=0.0}, {"frequency"=20.0, "amplitude"=0.1, "phase"=0.0}]) -> ("signal out"=w117:waveform(dbl))  [unwired: 6 in, 1 out]
            n29 = Unbundle By Name(w117) -> ("Y"=w118:dbl[])
          }
          frame 8 {
            # "SINE SWEEP"
            n30 = call <vilib>:"Chirp Pattern.vi"("f2"=0.5, "f1"=2.0, "amplitude"=1.0, "samples"=4500) -> ("Chirp Pattern"=w127:dbl[])  [unwired: 1 out]
            n31 = Multiply(x=w127, y=w121) -> (x*y=w126:dbl[])
            n32 = Add(x=w126, y=w121) -> (x+y=w125:dbl[])
            n33 = Array Subset(array=w125, index=38, length=256) -> (w122:dbl[])
          }
        }
        "SEQ1 Waveform" <- w51
        n34 = local read "RAM 1 SHAPE"() -> (w56:u16)
        n35 = To Unsigned Byte Integer(number=w51) -> (unsigned 8bit integer=w57:u8[])
        n36 = Bundle By Name(cluster=w59, "RAM 1 SHAPE"=w56, "RAM1"=w57) -> (w58:T1)
        n37 = Index Array(array=w60, index=w61) -> (element=w62:string)
      }
      frame "Build RAM2 Shape" {
        n38 = local read "RAM 2 SHAPE"() -> (w136:u16)
        n39 = Quotient & Remainder(x="RAM2 Peak", y=u8 2) -> (floor(x/y)=w134:u8)  [unwired: 1 out]
        n40 = case shown="7" w136 {
          tunnel: [w150 w154 w157 w165 w172 w180 w188 w199 w203] -> w137
          tunnel: "RAM2 Peak" -> [_ w153 w156 _ w171 w179 w187 _ _]
          tunnel: w134 -> [_ _ _ w164 _ _ _ w197 w202]
          frame 0, Default {
            # "ALL MIN"
            n41 = Initialize Array(u8 0, 256 ("dimension size")) -> (w150:u8[])
          }
          frame 1 {
            # "ALL MAX"
            n42 = Initialize Array(w153, 256 ("dimension size")) -> (w154:u8[])
          }
          frame 2 {
            # "SINE PULSE"
            n43 = call <vilib>:"Basic Function Generator.vi"("offset"=0.0, "sampling info"=cluster{"Fs":dbl, "#s":dbl} {"Fs"=256.0, "#s"=256.0}, "signal type"=T2."Sine Wave", "phase"=0.0, "amplitude"=w156, "frequency"=0.5) -> ("signal out"=w158:waveform(dbl))  [unwired: 3 in, 2 out]
            n44 = Unbundle By Name(w158) -> ("Y"=w157:dbl[])
          }
          frame 3 {
            # "HAVERSINE PULSE"
            n45 = call <vilib>:"Basic Function Generator.vi"("offset"=w164, "sampling info"=cluster{"Fs":dbl, "#s":dbl} {"Fs"=256.0, "#s"=256.0}, "signal type"=T2."Sine Wave", "phase"=270.0, "amplitude"=w164, "frequency"=1.0) -> ("signal out"=w166:waveform(dbl))  [unwired: 3 in, 2 out]
            n46 = Unbundle By Name(w166) -> ("Y"=w165:dbl[])
          }
          frame 4 {
            # "TRIANGLE PULSE"
            n47 = call <vilib>:"Basic Function Generator.vi"("offset"=0.0, "sampling info"=cluster{"Fs":dbl, "#s":dbl} {"Fs"=256.0, "#s"=256.0}, "signal type"=T2."Triangle Wave", "phase"=0.0, "amplitude"=w171, "frequency"=0.5) -> ("signal out"=w173:waveform(dbl))  [unwired: 3 in, 2 out]
            n48 = Unbundle By Name(w173) -> ("Y"=w172:dbl[])
          }
          frame 5 {
            # "POS RAMP"
            n49 = call <vilib>:"Basic Function Generator.vi"("offset"=0.0, "sampling info"=cluster{"Fs":dbl, "#s":dbl} {"Fs"=256.0, "#s"=256.0}, "signal type"=T2."Triangle Wave", "phase"=0.0, "amplitude"=w179, "frequency"=0.25) -> ("signal out"=w181:waveform(dbl))  [unwired: 3 in, 2 out]
            n50 = Unbundle By Name(w181) -> ("Y"=w180:dbl[])
          }
          frame 6 {
            # "NEG RAMP"
            n51 = call <vilib>:"Basic Function Generator.vi"("offset"=0.0, "sampling info"=cluster{"Fs":dbl, "#s":dbl} {"Fs"=256.0, "#s"=256.0}, "signal type"=T2."Triangle Wave", "phase"=90.0, "amplitude"=w187, "frequency"=0.25) -> ("signal out"=w189:waveform(dbl))  [unwired: 3 in, 2 out]
            n52 = Unbundle By Name(w189) -> ("Y"=w188:dbl[])
          }
          frame 7 {
            # "NOISE"
            n53 = Multiply(x=0.3125, y=w197) -> (x*y=w196:dbl)
            n54 = call <vilib>:"Tones and Noise Waveform.vi"("sampling info"=cluster{"Fs":dbl, "#s":dbl} {"Fs"=256.0, "#s"=256.0}, "offset"=w197, "noise (rms)"=w196, "tones"=T3 [{"frequency"=10.0, "amplitude"=0.0, "phase"=0.0}, {"frequency"=20.0, "amplitude"=0.1, "phase"=0.0}]) -> ("signal out"=w198:waveform(dbl))  [unwired: 6 in, 1 out]
            n55 = Unbundle By Name(w198) -> ("Y"=w199:dbl[])
          }
          frame 8 {
            # "SINE SWEEP"
            n56 = call <vilib>:"Chirp Pattern.vi"("f2"=0.5, "f1"=2.0, "amplitude"=1.0, "samples"=4500) -> ("Chirp Pattern"=w208:dbl[])  [unwired: 1 out]
            n57 = Multiply(x=w208, y=w202) -> (x*y=w207:dbl[])
            n58 = Add(x=w207, y=w202) -> (x+y=w206:dbl[])
            n59 = Array Subset(array=w206, index=38, length=256) -> (w203:dbl[])
          }
        }
        "SEQ2 Waveform" <- w137
        n60 = local read "RAM 2 SHAPE"() -> (w135:u16)
        n61 = To Unsigned Byte Integer(number=w137) -> (unsigned 8bit integer=w140:u8[])
        n62 = Bundle By Name(cluster=w139, "RAM 2 SHAPE"=w135, "RAM2"=w140) -> (w138:T1)
        n63 = Index Array(array=w141, index=w142) -> (element=w143:string)
      }
      frame "Downlink RAM1 Shape" {
        n64 = Unbundle By Name(w217) -> ("RAM1"=w215:u8[])
        n65 = for {
          N: 2 -> [_]
          shift-right: [w227] -> w213
          shift-left: w214 -> [w232]
          tunnel: w215 -> [w229]
          i -> [w236]
          w235 = u16 4 items=["Power UP", "Power DN", "Write Single", "Read Single", "Write Block", "Read Block", "Write Masked", "Test Value"] ("Function")
          w234 = u16 1 items=["Power ASIC", "Stim ASIC", "MICS Radio", "FRAM"] ("Target")
          n66 = case shown="1" w236 {
            tunnel: [u16 2048 ("SPI Address") u16 2176 ("SPI Address")] -> w231
            tunnel: [w240 w245] -> w230
            tunnel: w229 -> [w237 w242]
            frame 0, Default {
              n67 = Array Subset(array=w237, index=0, length=128) -> (w240:u8[])
            }
            frame 1 {
              n68 = Array Subset(array=w242, index=128, length=128) -> (w245:u8[])
            }
          }
          n69 = call "JTAG SPI.vi"("Block Write Data"=w230, "Blocksize"=i16 128 ("BlockSize"), "error in (no error)"=w232, "Target"=w234, "Function"=w235, "Address"=w231) -> ("error out"=w226:errorcluster)  [unwired: 2 in, 3 out]
          n70 = call "Simple Wait.vi"("mS"=u32 50, "error in"=w226) -> ("error out"=w227:errorcluster)  [unwired: 12 in, 1 out]
        }
        n71 = Index Array(array=w218, index=w219) -> (element=w220:string)
      }
      frame "Downlink RAM2 Shape" {
        n72 = Unbundle By Name(w251) -> ("RAM2"=w248:u8[])
        n73 = for {
          N: 2 -> [_]
          tunnel: w248 -> [w269]
          shift-right: [w267] -> w247
          shift-left: w249 -> [w263]
          i -> [w270]
          w260 = u16 1 items=["Power ASIC", "Stim ASIC", "MICS Radio", "FRAM"] ("Target")
          w261 = u16 4 items=["Power UP", "Power DN", "Write Single", "Read Single", "Write Block", "Read Block", "Write Masked", "Test Value"] ("Function")
          n74 = case shown="1" w270 {
            tunnel: [u16 2304 ("SPI Address") u16 2432 ("SPI Address")] -> w266
            tunnel: w269 -> [w274 w279]
            tunnel: [w273 w278] -> w262
            frame 0, Default {
              n75 = Array Subset(array=w274, index=0, length=128) -> (w273:u8[])
            }
            frame 1 {
              n76 = Array Subset(array=w279, index=128, length=128) -> (w278:u8[])
            }
          }
          n77 = call "JTAG SPI.vi"("Block Write Data"=w262, "Blocksize"=i16 128 ("BlockSize"), "error in (no error)"=w263, "Target"=w260, "Function"=w261, "Address"=w266) -> ("error out"=w264:errorcluster)  [unwired: 2 in, 3 out]
          n78 = call "Simple Wait.vi"("mS"=u32 50, "error in"=w264) -> ("error out"=w267:errorcluster)  [unwired: 12 in, 1 out]
        }
        n79 = Index Array(array=w252, index=w253) -> (element=w254:string)
      }
      frame "Downlink to UUT Finish" {
        w282 = u16 1 items=["Power ASIC", "Stim ASIC", "MICS Radio", "FRAM"] ("Target")
        w281 = u16 2 items=["Power UP", "Power DN", "Write Single", "Read Single", "Write Block", "Read Block", "Write Masked", "Test Value"] ("Function")
        n80 = Unbundle By Name(w290) -> ("Addresses"=w287:u16[], "Data"=w288:u8[])
        n81 = Unbundle By Name(w286) -> ("Downlink Progress"=w285:i32)
        n82 = Array Size(array=w287) -> (size(s)=w289:i32)
        n83 = while {
          shift-right: [w303] -> w283
          shift-left: w284 -> [w302]
          tunnel: w289 -> [w310]
          shift-right: [w309] -> _
          shift-left: w285 -> [w307]
          tunnel: w289 -> [w308]
          tunnel: w287 -> [w305]
          tunnel: w288 -> [w306]
          tunnel: w282 -> [w299]
          tunnel: w281 -> [w298]
          stop <- w311 stop-if-true
          n84 = Index Array(array=w305, index=w307) -> (element=w301:u16)
          n85 = Index Array(array=w306, index=w307) -> (element=w300:u8)
          n86 = Divide(x=w307, y=w308) -> (x/y=w304:dbl)
          n87 = local write "ProgBar"(w304) -> ()
          n88 = call "JTAG SPI.vi"("Value"=w300, "error in (no error)"=w302, "Target"=w299, "Function"=w298, "Address"=w301) -> ("error out"=w303:errorcluster)  [unwired: 3 in, 3 out]
          n89 = Increment(x=w307) -> (x+1=w309:i32)
          n90 = Greater Or Equal?(x=w309, y=w310) -> (x >= y?=w311:bool)
        }
        n91 = Index Array(array=w291, index=w292) -> (element=w293:string)
      }
      frame "Sync Panel" {
        w313 = 0
        w316 = FALSE
        n92 = local write "CONT"(w316) -> ()
        n93 = local write "RUN"(w316) -> ()
        n94 = local write "STOP"(w316) -> ()
        n95 = local write "SEL"(w316) -> ()
        n96 = local write "RST"(TRUE ("RST")) -> ()
        n97 = for {
          N: 4 -> [_]
          tunnel: [w325] -> w314 mode=indexing
          i -> [w326]
          n98 = case shown="3" w326 {
            tunnel: [w330 w334 w338 "Top of Loop"] -> w325
            frame 0, Default {
              n99 = Select(t="Apply Loads", s=FALSE, f="Open Loads") -> (s? t:f=w330:string)
            }
            frame 1 {
              n100 = Select(t="Short Caps", s=FALSE, f="Open Caps") -> (s? t:f=w334:string)
            }
            frame 2 {
              n101 = local read "Stop Clock"() -> (w335:bool)
              n102 = Select(t="Start CLK", s=w335, f="Stop CLK") -> (s? t:f=w338:string)
            }
            frame 3 {
            }
          }
        }
        n103 = Index Array(array=w314, index=w313) -> (element=w317:string)
      }
      frame "Start CLK" {
        n104 = call "JTAG Function.vi"("Enum"=T4."START_STIM_CLK", "error in (no error)"=w342) -> ("error out"=w341:errorcluster)  [unwired: 11 in, 2 out]
        n105 = Bundle By Name(cluster=w345, "Stop Clock"=TRUE) -> (w344:T1)
        n106 = Index Array(array=w347, index=w346) -> (element=w348:string)
      }
      frame "Stop CLK" {
        n107 = call "JTAG Function.vi"("Enum"=T4."STOP_STIM_CLK", "error in (no error)"=w356) -> ("error out"=w355:errorcluster)  [unwired: 11 in, 2 out]
        n108 = Bundle By Name(cluster=w359, "Stop Clock"=FALSE ("PHASE Changed")) -> (w358:T1)
        n109 = Index Array(array=w361, index=w360) -> (element=w362:string)
      }
      frame "Pulse Clock" {
        n110 = call "JTAG Function.vi"("Enum"=T4."PULSE_STIM_CLK", "ARG 1"="Pulses", "error in (no error)"=w371) -> ("error out"=w370:errorcluster)  [unwired: 10 in, 2 out]
        n111 = Index Array(array=w378, index=w377) -> (element=w379:string)
      }
      frame "Set STATE" {
        w401 = T9."Set Port Value" ("Function")
        n112 = local read "SEL"() -> (w399:bool)
        n113 = local read "STOP"() -> (w387:bool)
        n114 = local read "RUN"() -> (w386:bool)
        n115 = local read "CONT"() -> (w385:bool)
        n116 = local read "RST"() -> (w405:bool)
        n117 = Boolean To (0,1)(Boolean=w399) -> (0, 1=w400:i16)
        n118 = Boolean To (0,1)(Boolean=w387) -> (0, 1=w397:i16)
        n119 = Boolean To (0,1)(Boolean=w386) -> (0, 1=w395:i16)
        n120 = Boolean To (0,1)(Boolean=w385) -> (0, 1=w393:i16)
        n121 = Bundle By Name(cluster=w408, "SEL"=w399, "STOP"=w387, "RUN"=w386, "CONT"=w385, "RST"=w405) -> (w407:T1)
        n122 = Multiply(x=w400, y=u8 8) -> (x*y=w391:i16)
        n123 = Multiply(x=w397, y=u8 1) -> (x*y=w390:i16)
        n124 = Multiply(x=w395, y=u8 4) -> (x*y=w389:i16)
        n125 = Multiply(x=w393, y=u8 2) -> (x*y=w388:i16)
        n126 = Compound Arithmetic op=OR(w391, w390, w389, w388) -> (w384:i16)
        n127 = call "JTAG State.vi"("Quick Bit Function (Manual)"=T6."RST_N", "State (L)"=w405, "Function"=w401, "error in (no error)"=w406) -> ("error out"=w404:errorcluster)  [unwired: 9 in, 2 out]
        n128 = call "JTAG State.vi"("Quick Bit Function (Manual)"=T6."Manual Inputs", "Port (1)"=T5."Port 4", "Value (0)"=w384, "Mask (0)"=u8 15, "Function"=w401, "error in (no error)"=w404) -> ("error out"=w381:errorcluster)  [unwired: 7 in, 2 out]
        n129 = Index Array(array=w410, index=w409) -> (element=w411:string)
      }
      frame "Apply Loads" {
        w418 = TRUE  # Channel Loads:
        n130 = Bundle By Name(cluster=w420, "Channel Loads:"=w418) -> (w419:T1)
        n131 = Index Array(array=w422, index=w421) -> (element=w423:string)
      }
      frame "Open Loads" {
        w430 = FALSE  # Channel Loads:
        n132 = Bundle By Name(cluster=w432, "Channel Loads:"=w430) -> (w431:T1)
        n133 = Index Array(array=w434, index=w433) -> (element=w435:string)
      }
      frame "Short Caps" {
        w442 = TRUE  # Output Caps Shorted:
        n134 = Bundle By Name(cluster=w444, "Output Caps Shorted:"=w442) -> (w443:T1)
        n135 = Index Array(array=w446, index=w445) -> (element=w447:string)
      }
      frame "Open Caps" {
        w454 = FALSE  # Output Caps Shorted:
        n136 = Bundle By Name(cluster=w456, "Output Caps Shorted:"=w454) -> (w455:T1)
        n137 = Index Array(array=w458, index=w457) -> (element=w459:string)
      }
      frame "Init UUT" {
        w466 = u32 250 ("mS")
        w481 = TRUE  # UUT is UP
        n138 = call "JTAG Test Setup.vi"("error in (no error)"=w479, "BIT Value"=FALSE, "Test Function"=T7."PWR LDOA_EN BIT") -> ("error out"=w478:errorcluster)  [unwired: 8 in]
        n139 = call "Simple Wait.vi"("mS"=w466, "error in"=w478) -> ("error out"=w477:errorcluster)  [unwired: 12 in, 1 out]
        n140 = call "JTAG Function.vi"("Enum"=T4."STIM_POWER_DN", "error in (no error)"=w477) -> ("error out"=w480:errorcluster)  [unwired: 11 in, 2 out]
        n141 = call "Simple Wait.vi"("mS"=u32 1000, "error in"=w480) -> ("error out"=w469:errorcluster)  [unwired: 12 in, 1 out]
        n142 = call "JTAG Test Setup.vi"("error in (no error)"=w469, "BIT Value"=TRUE, "Test Function"=T7."PWR LDOA_EN BIT") -> ("error out"=w467:errorcluster)  [unwired: 8 in]
        n143 = call "Simple Wait.vi"("mS"=w466, "error in"=w467) -> ("error out"=w468:errorcluster)  [unwired: 12 in, 1 out]
        n144 = call "Saturn JTAG Startup.vi"("error in (no error)"=w468) -> ("error out"=w472:errorcluster)  [unwired: 14 in]
        n145 = call "Simple Wait.vi"("mS"=w466, "error in"=w472) -> ("error out"=w476:errorcluster)  [unwired: 12 in, 1 out]
        n146 = Bundle By Name(cluster=w483, "UUT is UP"=w481) -> (w482:T1)
        n147 = Index Array(array=w485, index=w484) -> (element=w486:string)
      }
      frame "Downlink to UUT" {
        w492 = 0
        # "Everything before the first phase register"
        n148 = Unbundle By Name(w512) -> ("Addresses"=w508:u16[], "Data"=w507:u8[])
        n149 = Array Size(array=w507) -> (size(s)=w509:i32)
        n150 = while {
          shift-right: [w566] -> w510
          shift-left: w513 -> [w567]
          tunnel: w508 -> [w565] mode=indexing
          tunnel: w507 -> [w564] mode=indexing
          tunnel: w509 -> [w579]
          tunnel: w508 -> [w578]
          tunnel: [w575] -> w505
          i -> [w575]
          stop <- w576 stop-if-true
          w562 = u16 2 items=["Power UP", "Power DN", "Write Single", "Read Single", "Write Block", "Read Block", "Write Masked", "Test Value"] ("Function")
          w563 = u16 1 items=["Power ASIC", "Stim ASIC", "MICS Radio", "FRAM"] ("Target")
          n151 = Increment(x=w575) -> (x+1=w577:i32)
          n152 = Index Array(array=w578, index=w577) -> (element=w571:u16)
          n153 = Divide(x=w575, y=w579) -> (x/y=w580:dbl)
          n154 = Equal?(x=u8 37, y=w565) -> (x = y?=w569:bool)
          n155 = local write "ProgBar"(w580) -> ()
          n156 = call "JTAG SPI.vi"("Value"=w564, "error in (no error)"=w567, "Target"=w563, "Function"=w562, "Address"=w565) -> ("error out"=w566:errorcluster)  [unwired: 3 in, 3 out]
          n157 = Select(t=u32 250 ("milliseconds to wait"), s=w569, f=u32 20 ("milliseconds to wait")) -> (s? t:f=w570:u32)
          n158 = Greater Or Equal?(x=w571, y=u8 64) -> (x >= y?=w576:bool)
          n159 = Wait (ms)(milliseconds to wait=w570) -> ()  [unwired: 1 out]
        }
        n160 = property on="ProgBar" class="Slide (strict)"("Caption.Text"="Send to UUT...") -> ()  [unwired: 2 in, 2 out]
        n161 = local read "Set RAM 1"() -> (w500:bool)
        n162 = Increment(x=w505) -> (x+1=w506:i32)
        n163 = while {
          shift-right: [w541] -> w502
          shift-left: w506 -> [w538]
          tunnel: w507 -> [w544]
          tunnel: w508 -> [w543]
          shift-right: [w533] -> w501
          shift-left: w510 -> [w534]
          tunnel: w509 -> [w539]
          i -> [w545]
          stop <- w540 stop-if-true
          w528 = u16 4 items=["Power UP", "Power DN", "Write Single", "Read Single", "Write Block", "Read Block", "Write Masked", "Test Value"] ("Function")
          w529 = u16 1 items=["Power ASIC", "Stim ASIC", "MICS Radio", "FRAM"] ("Target")
          n164 = Increment(x=w545) -> (x+1=w535:i32)
          n165 = Multiply(x=u8 64, y=w535) -> (x*y=w542:i32)
          n166 = while {
            tunnel: w544 -> [w560]
            tunnel: [w561] -> w531 mode=indexing
            tunnel: w543 -> [w558]
            tunnel: w542 -> [w547]
            tunnel: [w547] -> w530
            tunnel: [w553] -> w532
            shift-right: [w559] -> w541
            shift-left: w538 -> [w557]
            i -> [w554]
            stop <- w552 stop-if-true
            w548 = u8 64
            n167 = Increment(x=w557) -> (x+1=w556:i32)
            n168 = Increment(x=w557) -> (x+1=w559:i32)
            n169 = Add(x=w548, y=w547) -> (x+y=w555:i32)
            n170 = Index Array(array=w558, index=w556) -> (element=w549:u16)
            n171 = Index Array(array=w560, index=w557) -> (element=w561:u8)
            n172 = Increment(x=w554) -> (x+1=w553:i32)
            n173 = Greater Or Equal?(x=w549, y=w555) -> (x >= y?=w551:bool)
            n174 = Less?(x=w549, y=w548) -> (x < y?=w550:bool)
            n175 = Or(x=w551, y=w550) -> (x .or. y?=w552:bool)
          }
          n176 = Divide(x=w538, y=w539) -> (x/y=w537:dbl)
          n177 = local write "ProgBar"(w537) -> ()
          n178 = Greater Or Equal?(x=w535, y=24 ("x")) -> (x >= y?=w540:bool)
          n179 = call "JTAG SPI.vi"("Block Write Data"=w531, "Blocksize"=w532, "error in (no error)"=w534, "Target"=w529, "Function"=w528, "Address"=w530) -> ("error out"=w533:errorcluster)  [unwired: 2 in, 3 out]
          n180 = Wait (ms)(milliseconds to wait=u32 100) -> ()  [unwired: 1 out]
        }
        n181 = case shown="True" w500 {
          tunnel: string[] [] -> [w523 w525]
          tunnel: [w523 w526] -> w497
          frame False {
          }
          frame True {
            n182 = Build Array (concatenate)(w525, "Downlink RAM1 Shape") -> (w526:string[])
          }
        }
        n183 = local read "Set RAM 2"() -> (w498:bool)
        n184 = case shown="True" w498 {
          tunnel: w497 -> [w519 w521]
          tunnel: [w519 w522] -> w496
          frame False {
          }
          frame True {
            n185 = Build Array (concatenate)(w521, "Downlink RAM2 Shape") -> (w522:string[])
          }
        }
        n186 = Bundle By Name(cluster=w504, "Downlink Progress"=w502) -> (w503:T1)
        n187 = Build Array (concatenate)(w496, "Downlink to UUT Finish", "Top of Loop") -> (w493:string[])
        n188 = Index Array(array=w493, index=w492) -> (element=w514:string)
      }
      frame "Shutdown UUT" {
        w587 = FALSE  # UUT is UP
        # "NOTE power down AVDD as well"
        n189 = call "JTAG Test Setup.vi"("error in (no error)"=w585, "BIT Value"=FALSE, "Test Function"=T7."PWR LDOA_EN BIT") -> ("error out"=w584:errorcluster)  [unwired: 8 in]
        n190 = call "JTAG Function.vi"("Enum"=T4."STIM_POWER_DN", "error in (no error)"=w584) -> ("error out"=w586:errorcluster)  [unwired: 11 in, 2 out]
        n191 = Bundle By Name(cluster=w589, "UUT is UP"=w587) -> (w588:T1)
        n192 = Index Array(array=w591, index=w590) -> (element=w592:string)
      }
      frame "Build SPI" {
        w599 = u8[] []  # Data
        w598 = u16[] []  # Addresses
        n193 = Unbundle(w603) -> ("Set RAM 1"=w624:bool, "Set RAM 2"=w623:bool, "RAM 1 SHAPE"=w622:u16, "RAM 2 SHAPE"=w621:u16, "RECT 1"=w620:u8, "RECT 2"=w619:u8, "RECT 3"=w618:u8, "RECT 4"=w617:u8, "RECT 5"=w616:u8, "RECT 6"=w615:u8, "WaveDAC Ref Current"=w614:u8, "Set Basic Enables"=w613:bool, "Ph/Seq/Ram Wr Ena"=w612:bool, "Set WGE Bit"=w611:bool, "Set All RVLD Bits"=w610:bool, "Set PGOE Bit"=w609:bool, "Starting Phase 0"=w608:u8, "Ending Phase 0"=w607:u8, "Starting Phase 1"=w606:u8, "Ending Phase 1"=w605:u8, w604:T10)  [unwired: 2 out]
        n194 = while {
          shift-right: [w643] -> w600
          shift-left: w598 -> [w640]
          shift-right: [w642] -> w601
          shift-left: w599 -> [w639]
          tunnel: w624 -> [w664]
          tunnel: w623 -> [w663]
          tunnel: w622 -> [w662]
          tunnel: w621 -> [w661]
          tunnel: w620 -> [w660]
          tunnel: w619 -> [w659]
          tunnel: w618 -> [w658]
          tunnel: w617 -> [w657]
          tunnel: w616 -> [w656]
          tunnel: w615 -> [w655]
          tunnel: w614 -> [w654]
          tunnel: w613 -> [w653]
          tunnel: w612 -> [w652]
          tunnel: w611 -> [w651]
          tunnel: w610 -> [w650]
          tunnel: w609 -> [w649]
          tunnel: w608 -> [w648]
          tunnel: w607 -> [w647]
          tunnel: w606 -> [w646]
          tunnel: w605 -> [w645]
          tunnel: w604 -> [w644]
          tunnel: w599 -> [w638]
          tunnel: w598 -> [w637]
          i -> [w634]
          stop <- w665 stop-if-true
          n195 = To Unsigned Word Integer(number=w634) -> (unsigned 16bit integer=w641:u16)
          n196 = case shown="16" w641 {
            selector: w641 -> [_ w682 w701 w711 w721 w731 w741 w753 w769 w785 w801 w817 w832 w839 w846 w853 w860 w867 w874 w881 w888 w895 _ _ _ _ _ _ _]
            tunnel: [FALSE FALSE FALSE FALSE FALSE FALSE FALSE FALSE FALSE FALSE FALSE FALSE FALSE FALSE FALSE FALSE FALSE FALSE FALSE FALSE FALSE FALSE FALSE FALSE FALSE FALSE FALSE FALSE TRUE] -> w665
            tunnel: w640 -> [w667 w698 w708 w718 w728 w738 w748 w756 w772 w788 w804 w820 w835 w842 w849 w856 w863 w870 w877 w884 w891 w898 w906 w922 w937 w942 w960 w981 w1107]
            tunnel: w639 -> [w666 w697 w707 w717 w727 w737 w747 w755 w771 w787 w803 w819 w834 w841 w848 w855 w862 w869 w876 w883 w890 w897 w905 w923 w936 w943 w961 w978 w1106]
            tunnel: w664 -> [_ _ _ _ _ _ _ _ _ _ _ _ _ _ _ _ _ _ _ _ _ _ _ _ _ _ _ _ _]
            tunnel: w663 -> [_ _ _ _ _ _ _ _ _ _ _ _ _ _ _ _ _ _ _ _ _ _ _ _ _ _ _ _ _]
            tunnel: w662 -> [_ _ _ _ _ _ _ _ _ _ _ _ _ _ _ _ _ _ _ _ _ _ _ _ _ _ _ _ _]
            tunnel: w661 -> [_ _ _ _ _ _ _ _ _ _ _ _ _ _ _ _ _ _ _ _ _ _ _ _ _ _ _ _ _]
            tunnel: w660 -> [_ _ _ _ _ _ _ _ _ _ _ _ _ _ _ _ w859 _ _ _ _ _ _ _ _ _ _ _ _]
            tunnel: w659 -> [_ _ _ _ _ _ _ _ _ _ _ _ _ _ _ _ _ w866 _ _ _ _ _ _ _ _ _ _ _]
            tunnel: w658 -> [_ _ _ _ _ _ _ _ _ _ _ _ _ _ _ _ _ _ w873 _ _ _ _ _ _ _ _ _ _]
            tunnel: w657 -> [_ _ _ _ _ _ _ _ _ _ _ _ _ _ _ _ _ _ _ w880 _ _ _ _ _ _ _ _ _]
            tunnel: w656 -> [_ _ _ _ _ _ _ _ _ _ _ _ _ _ _ _ _ _ _ _ w887 _ _ _ _ _ _ _ _]
            tunnel: w655 -> [_ _ _ _ _ _ _ _ _ _ _ _ _ _ _ _ _ _ _ _ _ w894 _ _ _ _ _ _ _]
            tunnel: w654 -> [_ _ _ _ _ _ _ _ _ _ _ _ _ _ _ _ _ _ _ _ _ _ _ _ w933 _ _ _ _]
            tunnel: w653 -> [_ w695 _ _ _ _ _ _ _ _ _ _ _ _ _ _ _ _ _ _ _ _ _ _ _ _ _ _ _]
            tunnel: w652 -> [_ _ w703 w713 w723 w733 w743 _ _ _ _ _ _ _ _ _ _ _ _ _ _ _ _ _ _ _ _ _ w1105]
            tunnel: w651 -> [_ w694 _ _ _ _ _ _ _ _ _ _ _ _ _ _ _ _ _ _ _ _ _ _ _ _ _ _ _]
            tunnel: w650 -> [w671 _ _ _ _ _ _ w751 w767 w783 w799 w815 _ _ _ _ _ _ _ _ _ _ _ _ _ _ _ _ w1104]
            tunnel: w649 -> [_ w693 _ _ _ _ _ _ _ _ _ _ _ _ _ _ _ _ _ _ _ _ _ _ _ _ _ _ _]
            tunnel: w648 -> [_ _ _ _ _ _ _ _ _ _ _ _ w831 _ _ _ _ _ _ _ _ _ _ _ _ _ _ _ _]
            tunnel: w647 -> [_ _ _ _ _ _ _ _ _ _ _ _ _ w838 _ _ _ _ _ _ _ _ _ _ _ _ _ _ _]
            tunnel: w646 -> [_ _ _ _ _ _ _ _ _ _ _ _ _ _ w845 _ _ _ _ _ _ _ _ _ _ _ _ _ _]
            tunnel: w645 -> [_ _ _ _ _ _ _ _ _ _ _ _ _ _ _ w852 _ _ _ _ _ _ _ _ _ _ _ _ _]
            tunnel: w644 -> [_ _ _ _ _ _ _ _ _ _ _ _ _ _ _ _ _ _ _ _ _ _ _ _ _ _ _ w976 _]
            tunnel: [w669 w699 w709 w719 w729 w739 w749 w757 w773 w789 w805 w821 w836 w843 w850 w857 w864 w871 w878 w885 w892 w899 w907 w921 w938 w945 w959 w980 w1101] -> w643
            tunnel: [w668 w696 w706 w716 w726 w736 w746 w754 w770 w786 w802 w818 w833 w840 w847 w854 w861 w868 w875 w882 w889 w896 w904 w920 w935 w944 w958 w979 w1100] -> w642
            tunnel: w638 -> [_ _ _ _ _ _ _ _ _ _ _ _ _ _ _ _ _ _ _ _ _ _ _ _ _ _ _ w974 _]
            tunnel: w637 -> [_ _ _ _ _ _ _ _ _ _ _ _ _ _ _ _ _ _ _ _ _ _ _ _ _ _ _ w975 _]
            frame 0 {
              # "Pre-enable, allow writes to ENABLE and HV_CTL registers, optionally disable other bits"
              n197 = case shown="True" w671 {
                tunnel: [w673 w679] -> w669
                tunnel: [w672 w678] -> w668
                tunnel: w667 -> [w673 w677]
                tunnel: w666 -> [w672 w676]
                frame False {
                  # "Do not modify WE bits"
                }
                frame True {
                  w674 = u8[] [71]  # Data
                  w675 = u16[] [6]  # Addresses
                  n198 = Build Array (concatenate)(w677, w675) -> (w679:u16[])
                  n199 = Build Array (concatenate)(w676, w674) -> (w678:u8[])
                }
              }
            }
            frame 1, Default {
              # "ENABLE"
              # "PGOE"
              # "WGE"
              # "Basic Enables"
              n200 = property on="ProgBar" class="Slide (strict)"("Caption.Text"="Build SPI...") -> ()  [unwired: 2 in, 2 out]
              n201 = property on="ProgBar" class="Slide (strict)"("Visible"=TRUE) -> ()  [unwired: 2 in, 2 out]
              n202 = Select(t=u8 11, s=w695, f=u8 0) -> (s? t:f=w685:u8)
              n203 = Select(t=u8 4, s=w694, f=u8 0) -> (s? t:f=w686:u8)
              n204 = Select(t=u8 128, s=w693, f=u8 0) -> (s? t:f=w684:u8)
              n205 = Compound Arithmetic op=OR(w685, w686, w684) -> (w683:u8)
              n206 = Build Array (concatenate)(w698, w682) -> (w699:u16[])
              n207 = Build Array (concatenate)(w697, w683) -> (w696:u8[])
            }
            frame 2 {
              # "WE1"
              # "Write Enables"
              n208 = Select(t=u8 255, s=w703, f=u8 0) -> (s? t:f=w702:u8)
              n209 = Build Array (concatenate)(w708, w701) -> (w709:u16[])
              n210 = Build Array (concatenate)(w707, w702) -> (w706:u8[])
            }
            frame 3 {
              # "WE2"
              # "Write Enables"
              n211 = Select(t=u8 255, s=w713, f=u8 0) -> (s? t:f=w712:u8)
              n212 = Build Array (concatenate)(w718, w711) -> (w719:u16[])
              n213 = Build Array (concatenate)(w717, w712) -> (w716:u8[])
            }
            frame 4 {
              # "WE3"
              # "Write Enables"
              n214 = Select(t=u8 255, s=w723, f=u8 0) -> (s? t:f=w722:u8)
              n215 = Build Array (concatenate)(w728, w721) -> (w729:u16[])
              n216 = Build Array (concatenate)(w727, w722) -> (w726:u8[])
            }
            frame 5 {
              # "WE4"
              # "Write Enables"
              n217 = Select(t=u8 255, s=w733, f=u8 0) -> (s? t:f=w732:u8)
              n218 = Build Array (concatenate)(w738, w731) -> (w739:u16[])
              n219 = Build Array (concatenate)(w737, w732) -> (w736:u8[])
            }
            frame 6 {
              # "WE5"
              # "Write Enables"
              n220 = Select(t=u8 87, s=w743, f=u8 68) -> (s? t:f=w742:u8)
              n221 = Build Array (concatenate)(w748, w741) -> (w749:u16[])
              n222 = Build Array (concatenate)(w747, w742) -> (w746:u8[])
            }
            frame 7 {
              # "RVLD1"
              # "Set All RVLD Bits"
              n223 = case shown="True" w751 {
                tunnel: [w760 w766] -> w757
                tunnel: w756 -> [w760 w765]
                tunnel: w755 -> [w759 w764]
                tunnel: [w759 w763] -> w754
                tunnel: w753 -> [_ w762]
                tunnel: u8 0 -> [_ w761]
                frame False {
                }
                frame True {
                  n224 = Build Array (concatenate)(w765, w762) -> (w766:u16[])
                  n225 = Build Array (concatenate)(w764, w761) -> (w763:u8[])
                }
              }
            }
            frame 8 {
              # "RVLD2"
              # "Set All RVLD Bits"
              n226 = case shown="True" w767 {
                tunnel: [w776 w782] -> w773
                tunnel: w772 -> [w776 w781]
                tunnel: w771 -> [w775 w780]
                tunnel: [w775 w779] -> w770
                tunnel: w769 -> [_ w778]
                tunnel: u8 0 -> [_ w777]
                frame False {
                }
                frame True {
                  n227 = Build Array (concatenate)(w781, w778) -> (w782:u16[])
                  n228 = Build Array (concatenate)(w780, w777) -> (w779:u8[])
                }
              }
            }
            frame 9 {
              # "RVLD3"
              # "Set All RVLD Bits"
              n229 = case shown="True" w783 {
                tunnel: [w792 w798] -> w789
                tunnel: w788 -> [w792 w797]
                tunnel: w787 -> [w791 w796]
                tunnel: [w791 w795] -> w786
                tunnel: w785 -> [_ w794]
                tunnel: u8 0 -> [_ w793]
                frame False {
                }
                frame True {
                  n230 = Build Array (concatenate)(w797, w794) -> (w798:u16[])
                  n231 = Build Array (concatenate)(w796, w793) -> (w795:u8[])
                }
              }
            }
            frame 10 {
              # "RVLD4"
              # "Set All RVLD Bits"
              n232 = case shown="True" w799 {
                tunnel: [w808 w814] -> w805
                tunnel: w804 -> [w808 w813]
                tunnel: w803 -> [w807 w812]
                tunnel: [w807 w811] -> w802
                tunnel: w801 -> [_ w810]
                tunnel: u8 0 -> [_ w809]
                frame False {
                }
                frame True {
                  n233 = Build Array (concatenate)(w813, w810) -> (w814:u16[])
                  n234 = Build Array (concatenate)(w812, w809) -> (w811:u8[])
                }
              }
            }
            frame 11 {
              # "RVLD5"
              # "Set All RVLD Bits"
              n235 = case shown="True" w815 {
                tunnel: [w823 w830] -> w821
                tunnel: w820 -> [w823 w829]
                tunnel: w819 -> [w824 w828]
                tunnel: [w824 w827] -> w818
                tunnel: w817 -> [_ w826]
                tunnel: u8 0 -> [_ w825]
                frame False {
                }
                frame True {
                  n236 = Build Array (concatenate)(w829, w826) -> (w830:u16[])
                  n237 = Build Array (concatenate)(w828, w825) -> (w827:u8[])
                }
              }
            }
            frame 12 {
              # "SEQ0A"
              # "Starting Phase Sequence 0"
              n238 = Build Array (concatenate)(w835, w832) -> (w836:u16[])
              n239 = Build Array (concatenate)(w834, w831) -> (w833:u8[])
            }
            frame 13 {
              # "SEQ0B"
              # "Ending Phase Sequence 0"
              n240 = Build Array (concatenate)(w842, w839) -> (w843:u16[])
              n241 = Build Array (concatenate)(w841, w838) -> (w840:u8[])
            }
            frame 14 {
              # "SEQ1A"
              # "Starting Phase Sequence 1"
              n242 = Build Array (concatenate)(w849, w846) -> (w850:u16[])
              n243 = Build Array (concatenate)(w848, w845) -> (w847:u8[])
            }
            frame 15 {
              # "SEQ1B"
              # "Ending Phase Sequence 1"
              n244 = Build Array (concatenate)(w856, w853) -> (w857:u16[])
              n245 = Build Array (concatenate)(w855, w852) -> (w854:u8[])
            }
            frame 16 {
              # "RECT1"
              # "RECT 1 Amplitude"
              n246 = Build Array (concatenate)(w863, w860) -> (w864:u16[])
              n247 = Build Array (concatenate)(w862, w859) -> (w861:u8[])
            }
            frame 17 {
              # "RECT2"
              # "RECT 2 Amplitude"
              n248 = Build Array (concatenate)(w870, w867) -> (w871:u16[])
              n249 = Build Array (concatenate)(w869, w866) -> (w868:u8[])
            }
            frame 18 {
              # "RECT3"
              # "RECT 3 Amplitude"
              n250 = Build Array (concatenate)(w877, w874) -> (w878:u16[])
              n251 = Build Array (concatenate)(w876, w873) -> (w875:u8[])
            }
            frame 19 {
              # "RECT4"
              # "RECT 4 Amplitude"
              n252 = Build Array (concatenate)(w884, w881) -> (w885:u16[])
              n253 = Build Array (concatenate)(w883, w880) -> (w882:u8[])
            }
            frame 20 {
              # "RECT5"
              # "RECT 5 Amplitude"
              n254 = Build Array (concatenate)(w891, w888) -> (w892:u16[])
              n255 = Build Array (concatenate)(w890, w887) -> (w889:u8[])
            }
            frame 21 {
              # "RECT6"
              # "RECT 6 Amplitude"
              n256 = Build Array (concatenate)(w898, w895) -> (w899:u16[])
              n257 = Build Array (concatenate)(w897, w894) -> (w896:u8[])
            }
            frame 22 {
              # "BC_CTRL0"
              # "Boost Converter Programmed Voltage"
              n258 = case shown="True" TRUE {
                tunnel: [w910 w916] -> w907
                tunnel: w906 -> [w910 w915]
                tunnel: w905 -> [w909 w914]
                tunnel: [w909 w913] -> w904
                tunnel: "BC_CTRL0" -> [_ w912]
                tunnel: u16 32 ("SPI Address") -> [_ w911]
                frame False {
                }
                frame True {
                  n259 = Build Array (concatenate)(w915, w911) -> (w916:u16[])
                  n260 = Build Array (concatenate)(w914, w912) -> (w913:u8[])
                }
              }
            }
            frame 23 {
              # "BC_CTRL1"
              n261 = case shown="True" TRUE {
                tunnel: u16 33 ("SPI Address") -> [_ w932]
                tunnel: w923 -> [w925 w931]
                tunnel: "BC_CTRL1" -> [_ w930]
                tunnel: w922 -> [w926 w929]
                tunnel: [w926 w928] -> w921
                tunnel: [w925 w927] -> w920
                frame False {
                }
                frame True {
                  n262 = Build Array (concatenate)(w929, w932) -> (w928:u16[])
                  n263 = Build Array (concatenate)(w931, w930) -> (w927:u8[])
                }
              }
            }
            frame 24 {
              # "WFDAC"
              # "WaveDAC Ref Current"
              n264 = Build Array (concatenate)(w937, u16 37 ("SPI Address")) -> (w938:u16[])
              n265 = Build Array (concatenate)(w936, w933) -> (w935:u8[])
            }
            frame 25 {
              # "BG_CTRL"
              n266 = case shown="False" "BG_CTRL" {
                tunnel: u16 34 ("SPI Address") -> [_ w955]
                tunnel: [w949 w954] -> w945
                tunnel: [w948 w953] -> w944
                tunnel: w943 -> [w948 w952]
                tunnel: w942 -> [w949 w951]
                tunnel: "BG_CTRL 2" -> [_ w950]
                frame False {
                }
                frame True {
                  n267 = Build Array (concatenate)(w951, w955) -> (w954:u16[])
                  n268 = Build Array (concatenate)(w952, w950) -> (w953:u8[])
                }
              }
            }
            frame 26 {
              # "CG_CTRL"
              n269 = case shown="False" "CG_CTRL" {
                tunnel: u16 36 ("SPI Address") -> [_ w971]
                tunnel: "CG_CTRL 2" -> [_ w970]
                tunnel: w961 -> [w964 w969]
                tunnel: w960 -> [w965 w968]
                tunnel: [w965 w967] -> w959
                tunnel: [w964 w966] -> w958
                frame False {
                }
                frame True {
                  n270 = Build Array (concatenate)(w968, w971) -> (w967:u16[])
                  n271 = Build Array (concatenate)(w969, w970) -> (w966:u8[])
                }
              }
            }
            frame 27 {
              # "BUILD PHASE SEQUENCES"
              n272 = for {
                tunnel: w976 -> [w1058] mode=indexing
                shift-right: [w1055] -> w973
                shift-left: w975 -> [w1057]
                shift-right: [w1054] -> w972
                shift-left: w974 -> [w1056]
                tunnel: w975 -> [_]
                tunnel: w974 -> [_]
                i -> [w1048]
                w987 = u16[] [0, 1, 2, 3, 4, 5, 6, 7, 8]  # Addresses
                n273 = Unbundle(w1058) -> ("Enable"=w1053:bool[], "UCS/S"=w1052:bool[], "CBAL"=w1051:bool[], "Direction"=w1050:bool[], "Value"=w1049:u16[], "CAL"=w1043:bool[], "Waveform Source:"=w1042:u8, "Phase Repetitions:"=w1027:u8, "SYNC Sends:"=w1024:bool, "Delay/Pause Flag:"=w1033:bool, "Uncontrolled"=w1029:bool, "Clock Divider Enabled:"=w992:bool, "Clock Divisor(n+1):"=w996:u8, "STPC"=w1012:u8, "STPB+STPA"=w1013:u16, "PAUSE after PHASE:"=w1019:bool, "Trailing Delay(n+1CLK):"=w1006:u16, "Pulse Guard (n*128uS, 0=OFF)"=w998:u8, "Phase Offset:"=w1009:u8, "High Voltage is:"=w1035:bool)
                n274 = Not(x=w992) -> (.not. x?=w982:bool)
                n275 = Boolean To (0,1)(Boolean=w982) -> (0, 1=w991:i16)
                n276 = Multiply(x=w991, y=u8 128) -> (x*y=w990:i16)
                n277 = Boolean To (0,1)(Boolean=w1024) -> (0, 1=w1023:i16)
                n278 = Boolean To (0,1)(Boolean=w1029) -> (0, 1=w1028:i16)
                n279 = Boolean To (0,1)(Boolean=w1019) -> (0, 1=w1018:i16)
                n280 = To Unsigned Byte Integer(number=w990) -> (unsigned 8bit integer=w989:u8)
                n281 = Increment(x=w1048) -> (x+1=w1047:i32)
                n282 = Multiply(x=w1018, y=u8 16) -> (x*y=w1021:i16)
                n283 = Logical Shift(y=i16 -8, x=w1006) -> (x << y=w1007:u16)
                n284 = Not(x=w1035) -> (.not. x?=w983:bool)
                n285 = Multiply(x=u8 64, y=w1047) -> (x*y=w1045:i32)
                n286 = To Unsigned Byte Integer(number=w1006) -> (unsigned 8bit integer=w1005:u8)
                n287 = To Unsigned Byte Integer(number=w1007) -> (unsigned 8bit integer=w1004:u8)
                n288 = Compound Arithmetic op=OR(w996, w989) -> (w997:u8)
                n289 = To Unsigned Byte Integer(number=w1042) -> (unsigned 8bit integer=w1037:u8)
                n290 = Boolean To (0,1)(Boolean=w1033) -> (0, 1=w1031:i16)
                n291 = To Unsigned Byte Integer(number=w1027) -> (unsigned 8bit integer=w1026:u8)
                n292 = To Unsigned Byte Integer(number=w1021) -> (unsigned 8bit integer=w995:u8)
                n293 = Multiply(x=w1023, y=u8 16) -> (x*y=w1022:i16)
                n294 = To Unsigned Word Integer(number=w1045) -> (unsigned 16bit integer=w984:u16)
                n295 = Boolean To (0,1)(Boolean=w983) -> (0, 1=w1034:i16)
                n296 = To Unsigned Byte Integer(number=w1022) -> (unsigned 8bit integer=w994:u8)
                n297 = Multiply(x=w1031, y=u8 128) -> (x*y=w1041:i16)
                n298 = Multiply(x=w1028, y=u8 32) -> (x*y=w1040:i16)
                n299 = Multiply(x=u8 64, y=w1034) -> (x*y=w1039:i16)
                n300 = Logical Shift(y=i16 -8, x=w1013) -> (x << y=w1015:u16)
                n301 = Compound Arithmetic op=OR(w1026, w994, w995) -> (w993:u8)
                n302 = To Unsigned Byte Integer(number=w1013) -> (unsigned 8bit integer=w1017:u8)
                n303 = To Unsigned Byte Integer(number=w1015) -> (unsigned 8bit integer=w1014:u8)
                n304 = Compound Arithmetic op=OR(w1037, w1041, w1040, w1039) -> (w1038:i16)
                n305 = To Unsigned Byte Integer(number=w1038) -> (unsigned 8bit integer=w1010:u8)
                n306 = Build Array(w1010, w993, w1017, w1014, w1012, w1009, w1005, w1004, w997) -> (w1011:u8[])
                n307 = Add(x=w987, y=w984) -> (x+y=w986:u16[])
                n308 = Add(x=w984, y=u16 9) -> (x+y=w985:u16)
                n309 = for {
                  tunnel: w1053 -> [w1082] mode=indexing
                  tunnel: w1052 -> [w1083] mode=indexing
                  tunnel: w1051 -> [w1084] mode=indexing
                  tunnel: w1050 -> [w1085] mode=indexing
                  tunnel: w1049 -> [w1089] mode=indexing
                  tunnel: w985 -> [w1096]
                  shift-right: [w1093] -> w1003
                  shift-left: w986 -> [w1094]
                  shift-right: [w1091] -> w1000
                  shift-left: w1011 -> [w1062]
                  tunnel: w1043 -> [w1065] mode=indexing
                  tunnel: [w1059] -> w1001
                  i -> [w1099]
                  n310 = Boolean To (0,1)(Boolean=w1083) -> (0, 1=w1080:i16)
                  n311 = Boolean To (0,1)(Boolean=w1085) -> (0, 1=w1078:i16)
                  n312 = Boolean To (0,1)(Boolean=w1065) -> (0, 1=w1064:i16)
                  n313 = Logical Shift(y=i16 -8, x=w1089) -> (x << y=w1086:u16)
                  n314 = Boolean To (0,1)(Boolean=w1082) -> (0, 1=w1081:i16)
                  n315 = Boolean To (0,1)(Boolean=w1084) -> (0, 1=w1079:i16)
                  n316 = Multiply(x=w1099, y=u16 2) -> (x*y=w1097:i32)
                  n317 = To Unsigned Byte Integer(number=w1086) -> (unsigned 8bit integer=w1076:u8)
                  n318 = To Unsigned Byte Integer(number=w1089) -> (unsigned 8bit integer=w1090:u8)
                  n319 = To Unsigned Word Integer(number=w1097) -> (unsigned 16bit integer=w1095:u16)
                  n320 = Add(x=w1095, y=w1096) -> (x+y=w1092:u16)
                  n321 = Multiply(x=w1081, y=u8 16) -> (x*y=w1071:i16)
                  n322 = Multiply(x=w1080, y=u8 32) -> (x*y=w1072:i16)
                  n323 = Multiply(x=w1079, y=u8 64) -> (x*y=w1073:i16)
                  n324 = Multiply(x=w1078, y=u8 4) -> (x*y=w1074:i16)
                  n325 = Multiply(x=w1064, y=u8 128) -> (x*y=w1063:i16)
                  n326 = And(x=w1076, y=u8 3) -> (x .and. y?=w1077:u8)
                  n327 = Increment(x=w1092) -> (x+1=w1060:u16)
                  n328 = Compound Arithmetic op=OR(w1071, w1072, w1073, w1074, w1063, w1077) -> (w1087:i16)
                  n329 = Build Array (concatenate)(w1094, w1092, w1060) -> (w1093:u16[])
                  n330 = To Unsigned Byte Integer(number=w1087) -> (unsigned 8bit integer=w1061:u8)
                  n331 = Build Array (concatenate)(w1062, w1090, w1061) -> (w1091:u8[])
                  n332 = Increment(x=w1060) -> (x+1=w1059:u16)
                }
                n333 = Build Array (concatenate)(w1003, w1001) -> (w1002:u16[])
                n334 = Build Array (concatenate)(w1000, w998) -> (w999:u8[])
                n335 = Build Array (concatenate)(w1057, w1002) -> (w1055:u16[])
                n336 = Build Array (concatenate)(w1056, w999) -> (w1054:u8[])
              }
              n337 = Build Array (concatenate)(w981, w973) -> (w980:u16[])
              n338 = Build Array (concatenate)(w978, w972) -> (w979:u8[])
            }
            frame 28 {
              n339 = case shown="True" w1105 {
                tunnel: w1107 -> [w1118 w1124]
                tunnel: [w1118 w1123] -> w1102
                tunnel: [w1117 w1122] -> w1103
                tunnel: w1106 -> [w1117 w1121]
                frame False {
                  # "Do not modify Write Enable bits"
                }
                frame True {
                  w1120 = u8[] [0, 0, 0, 0, 84]  # Data
                  w1119 = u16[] [2, 3, 4, 5, 6]  # Addresses
                  # "Disable all WE Bits"
                  n340 = Build Array (concatenate)(w1124, w1119) -> (w1123:u16[])
                  n341 = Build Array (concatenate)(w1121, w1120) -> (w1122:u8[])
                }
              }
              n342 = case shown="True" w1104 {
                tunnel: w1102 -> [w1110 w1116]
                tunnel: [w1110 w1115] -> w1101
                tunnel: [w1109 w1114] -> w1100
                tunnel: w1103 -> [w1109 w1113]
                frame False {
                  # "Do not modify RVLD bits"
                }
                frame True {
                  w1112 = u8[] [255, 255, 255, 255, 3]  # Data
                  w1111 = u16[] [7, 8, 9, 10, 11]  # Addresses
                  # "Enable all RVLD Bits"
                  n343 = Build Array (concatenate)(w1116, w1111) -> (w1115:u16[])
                  n344 = Build Array (concatenate)(w1113, w1112) -> (w1114:u8[])
                }
              }
            }
          }
          n345 = Divide(x=w634, y=u8 26) -> (x/y=w636:dbl)
          n346 = local write "ProgBar"(w636) -> ()
        }
        n347 = Index Array(array=w626, index=w625) -> (element=w627:string)
        n348 = Bundle(cluster=w603, "Addresses"=w600, "Data"=w601) -> (w602:T11)  [unwired: 21 in]
      }
      frame "Save MAIN" {
        w1131 = "Select a Save Location"  # prompt
        w1132 = "Save"  # button label
        w1133 = "Saturn Phase Sequence Files"  # pattern label
        w1134 = "*.phf"  # pattern (all files)
        w1135 = "SaturnSequence.phf"  # default name
        n349 = call "File Dialog"("prompt"=w1131, "button label"=w1132, "default name"=w1135, "error in"=w1125, "pattern (all files)"=w1134, "pattern label"=w1133) -> ("selected path"=w1128:path, "cancelled"=w1130:bool, "error out"=w1129:errorcluster)  [unwired: 6 in, 1 out]
        n350 = case shown="False" w1130 {
          tunnel: w1129 -> [w1146 _]
          tunnel: w1128 -> [w1147 _]
          tunnel: [w1145 w1150] -> w1127
          tunnel: w1126 -> [w1144 _]
          tunnel: w1125 -> [_ w1150]
          frame False {
            n351 = Write to Binary File(file (use dialog)=w1147, data=w1144, error in=w1146) -> (refnum out=w1148:refnum<file>, error out=w1149:errorcluster)  [unwired: 3 in, 1 out]
            n352 = Close File(refnum=w1148, error in=w1149) -> (error out=w1145:errorcluster)  [unwired: 1 out]
          }
          frame True {
            w1151 = "Save was cancelled.  Data was not saved."  # message
            n353 = One Button Dialog(message=w1151) -> ()  [unwired: 1 in, 1 out]
          }
        }
        n354 = Index Array(array=w1137, index=w1136) -> (element=w1138:string)
      }
      frame "Load MAIN" {
        w1192 = "Select a Saturn Phase Sequence to Load"  # prompt
        w1193 = "Load"  # button label
        w1194 = "Saturn Phase Sequence Files"  # pattern label
        w1195 = "*.phf"  # pattern (all files)
        w1196 = "SaturnSequence.phf"  # default name
        n355 = call "File Dialog2"("prompt"=w1192, "button label"=w1193, "default name"=w1196, "error in"=w1154, "pattern (all files)"=w1195, "pattern label"=w1194) -> ("selected path"=w1189:path, "cancelled"=w1191:bool, "error out"=w1190:errorcluster)  [unwired: 6 in, 1 out]
        n356 = case shown="False" w1191 {
          tunnel: w1190 -> [w1202 _]
          tunnel: w1189 -> [w1207 _]
          tunnel: [w1202 w1209] -> w1188
          tunnel: w1153 -> [w1205 w1211]
          tunnel: [w1204 w1211] -> w1152
          tunnel: [w1201 w1210] -> w1186
          tunnel: w1154 -> [_ w1209]
          frame False {
            n357 = Read from Binary File(5:w1205, 8:w1202, 11:w1207) -> (0:w1203:errorcluster, 2:w1206:T11, 3:w1208:refnum<file>)  [unwired: 3 in, 1 out]
            n358 = Unbundle By Name(w1203) -> ("status"=w1201:bool)
            n359 = Close File(refnum=w1208, error in=w1203) -> ()  [unwired: 2 out]
            n360 = Select(t=w1205, s=w1201, f=w1206) -> (s? t:f=w1204:T11)
          }
          frame True {
            w1210 = TRUE  # status
            w1212 = "Load was cancelled.  Data was not changed."  # message
            n361 = One Button Dialog(message=w1212) -> ()  [unwired: 1 in, 1 out]
          }
        }
        n362 = Unbundle By Name(w1184) -> ("PHASE"=w1183:u8)
        n363 = Select(t=w1183, s=w1186, f=1) -> (s? t:f=w1179:i32)
        n364 = local write "PHASE"(w1179) -> ()
        n365 = Bundle By Name(cluster=w1184, "PHASE"=w1179) -> (w1187:T1)
        n366 = Unbundle(w1152) -> ("Set RAM 1"=w1155:bool, "Set RAM 2"=w1156:bool, "RAM 1 SHAPE"=w1157:u16, "RAM 2 SHAPE"=w1158:u16, "RECT 1"=w1161:u8, "RECT 2"=w1162:u8, "RECT 3"=w1163:u8, "RECT 4"=w1164:u8, "RECT 5"=w1165:u8, "RECT 6"=w1166:u8, "WaveDAC Ref Current"=w1167:u8, "Set Basic Enables"=w1168:bool, "Ph/Seq/Ram Wr Ena"=w1169:bool, "Set WGE Bit"=w1170:bool, "Set All RVLD Bits"=w1171:bool, "Set PGOE Bit"=w1172:bool, "Starting Phase 0"=w1173:u8, "Ending Phase 0"=w1174:u8, "Starting Phase 1"=w1175:u8, "Ending Phase 1"=w1176:u8, w1182:T10)  [unwired: 2 out]
        n367 = Decrement(x=w1179) -> (x-1=w1180:i32)
        n368 = Index Array(array=w1182, index=w1180) -> (element=w1181:T8)
        n369 = Bundle(cluster=w1178, "RECT 1"=w1161, "RECT 2"=w1162, "RECT 3"=w1163, "RECT 4"=w1164, "RECT 5"=w1165, "RECT 6"=w1166, "WaveDAC Ref Current"=w1167, "Set Basic Enables"=w1168, "Ph/Seq/Ram Wr Ena"=w1169, "Set WGE Bit"=w1170, "Set All RVLD Bits"=w1171, "Set PGOE Bit"=w1172, "Starting Phase 0"=w1173, "Ending Phase 0"=w1174, "Starting Phase 1"=w1175, "Ending Phase 1"=w1176) -> (w1177:T12)
        n370 = Bundle(cluster=w1160, "Set RAM 1"=w1155, "Set RAM 2"=w1156, "RAM 1 SHAPE"=w1157, "RAM 2 SHAPE"=w1158) -> (w1159:T13)
        n371 = Index Array(array=w1198, index=w1197) -> (element=w1199:string)
      }
      frame "Change PHASE" {
        n372 = Unbundle(w1215) -> (w1222:T10)  [unwired: 22 out]
        n373 = local read "PHASE"() -> (w1213:u8)
        n374 = Decrement(x=w1213) -> (x-1=w1214:u8)
        n375 = Index Array(array=w1222, index=w1214) -> (element=w1221:T8)
        n376 = Bundle By Name(cluster=w1220, "PHASE"=w1213) -> (w1219:T1)
        n377 = Index Array(array=w1217, index=w1216) -> (element=w1218:string)
      }
      frame "Top of Loop" {
        w1236 = u32 10  # milliseconds to wait
        w1257 = u8 0
        n378 = Unbundle By Name(w1239) -> ("UUT is UP"=w1229:bool)
        "ACTIVE" <- w1229
        n379 = property on="ProgBar" class="Slide (strict)"("Visible"=FALSE) -> ()  [unwired: 2 in, 2 out]
        n380 = case shown="\"Stim\"" "Tab Control" {
          tunnel: string[] ["Top of Loop"] -> [w1268 w1274]
          tunnel: [w1268 w1273] -> w1243
          tunnel: w1229 -> [_ w1271]
          tunnel: [w1267 w1270] -> w1242
          tunnel: w1239 -> [w1267 w1269]
          frame "General", Default {
            # "General Control Page"
          }
          frame "Stim" {
            # "Stim ASIC Control Page"
            # "Process User Commands"
            n381 = for {
              N: 13 -> [_]
              shift-right: [w1279] -> w1273
              shift-left: w1274 -> [w1280]
              tunnel: w1271 -> [w1278]
              tunnel: w1269 -> [w1277]
              tunnel: [w1275] -> w1270
              tunnel: w1269 -> [w1276]
              i -> [w1281]
              n382 = case shown="2" w1281 {
                tunnel: w1280 -> [w1285 w1291 w1303 w1308 w1311 w1317 w1319 w1339 w1351 w1359 w1366 w1374 w1385]
                tunnel: [w1284 w1290 w1302 w1307 w1310 w1316 w1319 w1340 w1352 w1359 w1367 w1373 w1386] -> w1279
                tunnel: w1278 -> [_ w1289 _ _ _ _ _ _ _ _ _ _ _]
                tunnel: w1277 -> [_ _ _ _ _ _ _ w1325 w1348 _ w1363 w1371 w1384]
                tunnel: w1276 -> [w1282 w1287 w1299 w1304 w1309 w1314 w1320 w1321 w1343 w1360 w1361 w1370 w1381]
                tunnel: [w1282 w1287 w1299 w1304 w1309 w1314 w1320 w1321 w1343 w1360 w1361 w1370 w1380] -> w1275
                frame 0, Default {
                  n383 = Select(t=string[] ["Clear MAIN", "Write BASE", "Write SEQ", "Write PHASE", "Top of Loop"], s="Clear", f=w1285) -> (s? t:f=w1284:string[])
                }
                frame 1 {
                  n384 = case shown="False" w1289 {
                    tunnel: w1291 -> [w1292 w1298]
                    tunnel: [w1292 w1297] -> w1290
                    tunnel: "Download" -> [w1293 w1295]
                    frame False {
                      n385 = case shown="True" w1293 {
                        frame False {
                        }
                        frame True {
                          n386 = One Button Dialog(message="UUT is not running.  Use \"Reset UUT\"\nto bring it online before downlinking!") -> ()  [unwired: 1 in, 1 out]
                        }
                      }
                    }
                    frame True {
                      n387 = Select(t=string[] ["Read PHASE", "Read BASE", "Read SEQ", "Build SPI", "Downlink to UUT"], s=w1295, f=w1298) -> (s? t:f=w1297:string[])
                    }
                  }
                }
                frame 2 {
                  n388 = Select(t=string[] ["Init UUT", "Sync Panel"], s="Reset", f=w1303) -> (s? t:f=w1302:string[])
                }
                frame 3 {
                  n389 = Select(t=string[] ["Read BASE", "Read SEQ", "Read PHASE", "Load MAIN", "Write PHASE", "Write SEQ", "Write BASE", "Top of Loop"], s="Load", f=w1308) -> (s? t:f=w1307:string[])
                }
                frame 4 {
                  n390 = Select(t=string[] ["Read PHASE", "Read BASE", "Read SEQ", "Build SPI", "Save MAIN", "Top of Loop"], s="Save", f=w1311) -> (s? t:f=w1310:string[])
                }
                frame 5 {
                  n391 = Select(t=string[] ["Shutdown UUT", "Top of Loop"], s="Shutdown UUT", f=w1317) -> (s? t:f=w1316:string[])
                }
                frame 6 {
                }
                frame 7 {
                  n392 = Unbundle By Name(w1325) -> ("CONT"=w1334:bool)
                  n393 = Unbundle By Name(w1325) -> ("RUN"=w1338:bool)
                  n394 = Unbundle By Name(w1325) -> ("STOP"=w1329:bool)
                  n395 = Unbundle By Name(w1325) -> ("SEL"=w1331:bool)
                  n396 = Unbundle By Name(w1325) -> ("RST"=w1323:bool)
                  n397 = Exclusive Or(1:w1334, 2:"CONT") -> (0:w1332:bool)
                  n398 = Exclusive Or(1:w1338, 2:"RUN") -> (0:w1335:bool)
                  n399 = Exclusive Or(1:w1329, 2:"STOP") -> (0:w1327:bool)
                  n400 = Exclusive Or(1:w1331, 2:"SEL") -> (0:w1326:bool)
                  n401 = Exclusive Or(1:w1323, 2:"RST") -> (0:w1322:bool)
                  n402 = Compound Arithmetic op=OR(w1332, w1335, w1327, w1326, w1322) -> (w1336:bool)
                  n403 = case shown="True" w1336 {
                    tunnel: [w1341 string[] ["Set STATE", "Top of Loop"]] -> w1340
                    tunnel: w1339 -> [w1341 _]
                    frame False {
                    }
                    frame True {
                    }
                  }
                }
                frame 8 {
                  w1346 = T14."Enabled"  # Disabled
                  w1347 = T14."Disabled and Grayed Out"  # Disabled
                  n404 = Unbundle By Name(w1348) -> ("Stop Clock"=w1349:bool)
                  n405 = Exclusive Or(1:w1349, 2:"Stop Clock") -> (0:w1350:bool)
                  n406 = case shown="True" w1350 {
                    tunnel: [w1353 w1356] -> w1352
                    tunnel: w1351 -> [w1353 w1355]
                    tunnel: "Stop Clock" -> [_ w1354]
                    frame False {
                    }
                    frame True {
                      n407 = case shown="False" w1354 {
                        tunnel: w1355 -> [_ _]
                        tunnel: [string[] ["Start CLK", "Top of Loop"] string[] ["Stop CLK", "Top of Loop"]] -> w1356
                        frame True {
                        }
                        frame False {
                        }
                      }
                    }
                  }
                  n408 = Select(t=w1347, s="Stop Clock", f=w1346) -> (s? t:f=w1344:T14)
                  n409 = property on="Pulse Clock" class="Bool (strict)"("DisabledEnum"=w1344) -> ()  [unwired: 2 in, 2 out]
                }
                frame 9 {
                }
                frame 10 {
                  n410 = local read "RAM 1 SHAPE"() -> (w1362:u16)
                  n411 = Unbundle By Name(w1363) -> ("RAM 1 SHAPE"=w1364:u16)
                  n412 = Not Equal?(x=w1362, y=w1364) -> (x != y?=w1365:bool)
                  n413 = case shown="True" w1365 {
                    tunnel: [w1368 string[] ["Build RAM1 Shape", "Top of Loop"]] -> w1367
                    tunnel: w1366 -> [w1368 _]
                    frame False {
                    }
                    frame True {
                    }
                  }
                }
                frame 11 {
                  n414 = local read "RAM 2 SHAPE"() -> (w1372:u16)
                  n415 = Unbundle By Name(w1371) -> ("RAM 2 SHAPE"=w1375:u16)
                  n416 = Not Equal?(x=w1372, y=w1375) -> (x != y?=w1376:bool)
                  n417 = case shown="True" w1376 {
                    tunnel: [w1377 string[] ["Build RAM2 Shape", "Top of Loop"]] -> w1373
                    tunnel: w1374 -> [w1377 _]
                    frame False {
                    }
                    frame True {
                    }
                  }
                }
                frame 12 {
                  n418 = Unbundle By Name(w1384) -> ("Pulse"=w1382:bool)
                  n419 = Greater?(x="Pulse Clock", y=w1382) -> (0:w1383:bool)
                  n420 = case shown="False" w1383 {
                    tunnel: [w1390 string[] ["Pulse Clock", "Top of Loop"]] -> w1386
                    tunnel: w1385 -> [w1390 _]
                    tunnel: w1381 -> [w1389 w1395]
                    tunnel: [w1388 w1395] -> w1380
                    tunnel: "Pulse Clock" -> [w1387 _]
                    frame False {
                      n421 = case shown="True" w1387 {
                        selector: w1387 -> [w1391 _]
                        tunnel: w1389 -> [w1393 w1394]
                        tunnel: [w1392 w1394] -> w1388
                        frame False {
                          n422 = Bundle By Name(cluster=w1393, "Pulse"=w1391) -> (w1392:T1)
                        }
                        frame True {
                        }
                      }
                    }
                    frame True {
                    }
                  }
                }
              }
            }
          }
        }
        n423 = Wait (ms)(milliseconds to wait=w1236) -> ()  [unwired: 1 out]
        n424 = And(x=w1229, y="Status Polling") -> (x .and. y?=w1227:bool)
        n425 = case shown="True" w1227 {
          tunnel: [w1397 w1410] -> w1253
          tunnel: [w1397 u8 0 ("Single Read")] -> _
          tunnel: [TRUE ("Quick Bit Read") w1406] -> w1237
          tunnel: [w1397 w1402] -> w1233
          frame False {
            w1397 = u8 0  # Single Read
          }
          frame True {
            w1399 = u16 1 items=["Power ASIC", "Stim ASIC", "MICS Radio", "FRAM"] ("Target")
            w1400 = u16 3 items=["Power UP", "Power DN", "Write Single", "Read Single", "Write Block", "Read Block", "Write Masked", "Test Value"] ("Function")
            w1405 = u32 200  # milliseconds to wait
            n426 = Wait (ms)(milliseconds to wait=w1405) -> ()  [unwired: 1 out]
            n427 = call "JTAG SPI.vi"("Target"=w1399, "Function"=w1400, "Address"=u16 0) -> ("error out"=w1408:errorcluster, "Read Value"=w1410:u8)  [unwired: 5 in, 2 out]
            n428 = call "JTAG State.vi"("Quick Bit Function (Manual)"=T6."STIM_ERR (IN)", "error in (no error)"=w1408) -> ("Quick Bit Read"=w1406:bool, "error out"=w1404:errorcluster)  [unwired: 11 in, 1 out]
            n429 = call "JTAG State.vi"("Port (1)"=T5."Port 4", "error in (no error)"=w1404) -> ("Manual Read"=w1402:u8)  [unwired: 11 in, 2 out]
          }
        }
        n430 = Number To Boolean Array(number=w1253) -> (Boolean array=w1254:bool[])
        n431 = Number To Boolean Array(number=w1233) -> (Boolean array=w1235:bool[])
        n432 = Array To Cluster(array=w1254) -> (cluster=w1252:T15)
        n433 = Array To Cluster(array=w1235) -> (cluster=w1234:T15)
        n434 = Unbundle By Name(w1252) -> ("Boolean array[5]"=→"WPF":bool, "Boolean array[0]"=→"PGF":bool, "Boolean array[1]"=→"PARF":bool, "Boolean array[2]"=→"SEQF":bool, "Boolean array[3]"=→"ADRF":bool, "Boolean array[4]"=→"RVF":bool)
        n435 = Unbundle By Name(w1234) -> ("Boolean array[6]"=→"PROG":bool, "Boolean array[5]"=→"PAUSE":bool, "Boolean array[4]"=→"SYNC":bool)
        n436 = Not(x=w1237) -> (.not. x?=→"ERR_N":bool)
        n437 = Unbundle By Name(w1242) -> ("PHASE"=w1261:u8)
        n438 = Not Equal?(x="PHASE", y=w1261) -> (x != y?=w1260:bool)
        n439 = Select(t=string[] ["Read PHASE", "Change PHASE", "Write PHASE", "Top of Loop"], s=w1260, f=w1243) -> (s? t:f=w1258:string[])
        n440 = Index Array(array=w1258, index=w1257) -> (element=w1256:string)
      }
      frame "Build MAIN" {
        w1411 = 1
        w1420 = FALSE
        w1427 = u8[] []  # Data
        w1428 = u16[] []  # Addresses
        n441 = local read "STOP"() -> (w1416:bool)
        n442 = local read "RUN"() -> (w1417:bool)
        n443 = local read "CONT"() -> (w1418:bool)
        n444 = local read "SEL"() -> (w1419:bool)
        n445 = Unbundle(w1450) -> ("Set RAM 1"=w1448:bool, "Set RAM 2"=w1447:bool, "RAM 1 SHAPE"=w1446:u16, "RAM 2 SHAPE"=w1445:u16)
        n446 = Unbundle(w1449) -> ("RECT 1"=w1444:u8, "RECT 2"=w1443:u8, "RECT 3"=w1442:u8, "RECT 4"=w1441:u8, "RECT 5"=w1440:u8, "RECT 6"=w1439:u8, "WaveDAC Ref Current"=w1438:u8, "Set Basic Enables"=w1437:bool, "Ph/Seq/Ram Wr Ena"=w1436:bool, "Set WGE Bit"=w1435:bool, "Set All RVLD Bits"=w1434:bool, "Set PGOE Bit"=w1433:bool, "Starting Phase 0"=w1432:u8, "Ending Phase 0"=w1431:u8, "Starting Phase 1"=w1430:u8, "Ending Phase 1"=w1429:u8)
        n447 = local write "PHASE"(w1411) -> ()
        n448 = Initialize Array(w1423, 24 ("dimension size")) -> (w1424:T10)
        n449 = Bundle By Name(cluster=w1422, "PHASE Changed"=w1420, "BASE Changed"=w1420, "SEQ Changed"=TRUE, "PHASE"=w1411, "STOP"=w1416, "RUN"=w1417, "CONT"=w1418, "SEL"=w1419) -> (w1421:T1)
        n450 = Bundle("Set RAM 1"=w1448, "Set RAM 2"=w1447, "RAM 1 SHAPE"=w1446, "RAM 2 SHAPE"=w1445, "RECT 1"=w1444, "RECT 2"=w1443, "RECT 3"=w1442, "RECT 4"=w1441, "RECT 5"=w1440, "RECT 6"=w1439, "WaveDAC Ref Current"=w1438, "Set Basic Enables"=w1437, "Ph/Seq/Ram Wr Ena"=w1436, "Set WGE Bit"=w1435, "Set All RVLD Bits"=w1434, "Set PGOE Bit"=w1433, "Starting Phase 0"=w1432, "Ending Phase 0"=w1431, "Starting Phase 1"=w1430, "Ending Phase 1"=w1429, w1424, "Addresses"=w1428, "Data"=w1427) -> (w1425:T11)  [unwired: 1 in]
        n451 = Index Array(array=w1412, index=w1413) -> (element=w1414:string)
      }
      frame "Read BASE" {
        n452 = Bundle("RECT 1"="RECT 1", "RECT 2"="RECT 2", "RECT 3"="RECT 3", "RECT 4"="RECT 4", "RECT 5"="RECT 5", "RECT 6"="RECT 6", "WFD_CTRL"="WFD_CTRL", "Set Basic Enables"="Set Basic Enables", "Ph/Seq/Ram Wr Ena"="Ph/Seq/Ram Wr Ena", "Set WGE Bit"="Set WGE Bit", "Set All RVLD Bits"="Set All RVLD Bits", "Set PGOE Bit"="Set PGOE Bit", "Starting Phase 0"="Starting Phase 0", "Ending Phase 0"="Ending Phase 0", "Starting Phase 1"="Starting Phase 1", "Ending Phase 1"="Ending Phase 1") -> (w1475:T16)  [unwired: 1 in]
        n453 = Bundle(cluster=w1470, "RECT 1"="RECT 1", "RECT 2"="RECT 2", "RECT 3"="RECT 3", "RECT 4"="RECT 4", "RECT 5"="RECT 5", "RECT 6"="RECT 6", "WaveDAC Ref Current"="WFD_CTRL", "Set Basic Enables"="Set Basic Enables", "Ph/Seq/Ram Wr Ena"="Ph/Seq/Ram Wr Ena", "Set WGE Bit"="Set WGE Bit", "Set All RVLD Bits"="Set All RVLD Bits", "Set PGOE Bit"="Set PGOE Bit", "Starting Phase 0"="Starting Phase 0", "Ending Phase 0"="Ending Phase 0", "Starting Phase 1"="Starting Phase 1", "Ending Phase 1"="Ending Phase 1") -> (w1469:T11)  [unwired: 7 in]
        n454 = Index Array(array=w1472, index=w1471) -> (element=w1473:string)
      }
      frame "Write BASE" {
        n455 = Unbundle By Name(w1500) -> ("RECT 1"=w1484:u8, "RECT 2"=w1485:u8, "RECT 3"=w1486:u8, "RECT 4"=w1487:u8, "RECT 5"=w1488:u8, "RECT 6"=w1489:u8, "WaveDAC Ref Current"=w1490:u8, "Set Basic Enables"=w1491:bool, "Ph/Seq/Ram Wr Ena"=w1492:bool, "Set WGE Bit"=w1493:bool, "Set All RVLD Bits"=w1494:bool, "Set PGOE Bit"=w1495:bool, "Starting Phase 0"=w1496:u8, "Ending Phase 0"=w1497:u8, "Starting Phase 1"=w1498:u8, "Ending Phase 1"=w1499:u8)
        n456 = local write "RECT 1"(w1484) -> ()
        n457 = local write "RECT 2"(w1485) -> ()
        n458 = local write "RECT 3"(w1486) -> ()
        n459 = local write "RECT 4"(w1487) -> ()
        n460 = local write "RECT 5"(w1488) -> ()
        n461 = local write "RECT 6"(w1489) -> ()
        n462 = local write "WFD_CTRL"(w1490) -> ()
        n463 = local write "Set Basic Enables"(w1491) -> ()
        n464 = local write "Ph/Seq/Ram Wr Ena"(w1492) -> ()
        n465 = local write "Set WGE Bit"(w1493) -> ()
        n466 = local write "Set All RVLD Bits"(w1494) -> ()
        n467 = local write "Set PGOE Bit"(w1495) -> ()
        n468 = local write "Starting Phase 0"(w1496) -> ()
        n469 = local write "Ending Phase 0"(w1497) -> ()
        n470 = local write "Starting Phase 1"(w1498) -> ()
        n471 = local write "Ending Phase 1"(w1499) -> ()
        n472 = Index Array(array=w1481, index=w1480) -> (element=w1482:string)
      }
      frame "Init" {
        w1508 = u8 0
        w1509 = string[] ["Read BASE", "Read PHASE", "Read SEQ", "Build MAIN", "Top of Loop"]
        n473 = Bundle By Name(cluster=w1512, "Override Changes"=TRUE) -> (w1511:T1)
        n474 = Index Array(array=w1509, index=w1508) -> (element=w1507:string)
      }
      frame "Read PHASE" {
        n475 = for {
          N: 26 -> [_]
          tunnel: [w1563] -> w1544 mode=indexing
          tunnel: [w1562] -> w1545 mode=indexing
          tunnel: [w1561] -> w1546 mode=indexing
          tunnel: [w1560] -> w1547 mode=indexing
          tunnel: [w1559] -> w1548 mode=indexing
          tunnel: [w1558] -> w1549 mode=indexing
          i -> [w1564]
          n476 = case shown="25" w1564 {
            tunnel: ["Cal 1" "Cal 2" "Cal 3" "Cal 4" "Cal 5" "Cal 6" "Cal 7" "Cal 8" "Cal 9" "Cal 10" "Cal 11" "Cal 12" "Cal 13" "Cal 14" "Cal 15" "Cal 16" "Cal 17" "Cal 18" "Cal 19" "Cal 20" "Cal 21" "Cal 22" "Cal 23" "Cal 24" "Cal 25" "Cal 26"] -> w1563
            tunnel: ["Value Ch 1" "Value Ch 2" "Value Ch 3" "Value Ch 4" "Value Ch 5" "Value Ch 6" "Value Ch 7" "Value Ch 8" "Value Ch 9" "Value Ch 10" "Value Ch 11" "Value Ch 12" "Value Ch 13" "Value Ch 14" "Value Ch 15" "Value Ch 16" "Value Ch 17" "Value Ch 18" "Value Ch 19" "Value Ch 20" "Value Ch 21" "Value Ch 22" "Value Ch 23" "Value Ch 24" "Value Ch 25" "Value Ch 26"] -> w1562
            tunnel: ["Direction 1" "Direction 2" "Direction 3" "Direction 4" "Direction 5" "Direction 6" "Direction 7" "Direction 8" "Direction 9" "Direction 10" "Direction 11" "Direction 12" "Direction 13" "Direction 14" "Direction 15" "Direction 16" "Direction 17" "Direction 18" "Direction 19" "Direction 20" "Direction 21" "Direction 22" "Direction 23" "Direction 24" "Direction 25" "Direction 26"] -> w1561
            tunnel: ["CBAL 1" "CBAL 2" "CBAL 3" "CBAL 4" "CBAL 5" "CBAL 6" "CBAL 7" "CBAL 8" "CBAL 9" "CBAL 10" "CBAL 11" "CBAL 12" "CBAL 13" "CBAL 14" "CBAL 15" "CBAL 16" "CBAL 17" "CBAL 18" "CBAL 19" "CBAL 20" "CBAL 21" "CBAL 22" "CBAL 23" "CBAL 24" "CBAL 25" "CBAL 26"] -> w1560
            tunnel: ["UCS/S 1" "UCS/S 2" "UCS/S 3" "UCS/S 4" "UCS/S 5" "UCS/S 6" "UCS/S 7" "UCS/S 8" "UCS/S 9" "UCS/S 10" "UCS/S 11" "UCS/S 12" "UCS/S 13" "UCS/S 14" "UCS/S 15" "UCS/S 16" "UCS/S 17" "UCS/S 18" "UCS/S 19" "UCS/S 20" "UCS/S 21" "UCS/S 22" "UCS/S 23" "UCS/S 24" "UCS/S 25" "UCS/S 26"] -> w1559
            tunnel: ["Enable 1" "Enable 2" "Enable 3" "Enable 4" "Enable 5" "Enable 6" "Enable 7" "Enable 8" "Enable 9" "Enable 10" "Enable 11" "Enable 12" "Enable 13" "Enable 14" "Enable 15" "Enable 16" "Enable 17" "Enable 18" "Enable 19" "Enable 20" "Enable 21" "Enable 22" "Enable 23" "Enable 24" "Enable 25" "Enable 26"] -> w1558
            frame 0, Default {
            }
            frame 1 {
            }
            frame 2 {
            }
            frame 3 {
            }
            frame 4 {
            }
            frame 5 {
            }
            frame 6 {
            }
            frame 7 {
            }
            frame 8 {
            }
            frame 9 {
            }
            frame 10 {
            }
            frame 11 {
            }
            frame 12 {
            }
            frame 13 {
            }
            frame 14 {
            }
            frame 15 {
            }
            frame 16 {
            }
            frame 17 {
            }
            frame 18 {
            }
            frame 19 {
            }
            frame 20 {
            }
            frame 21 {
            }
            frame 22 {
            }
            frame 23 {
            }
            frame 24 {
            }
            frame 25 {
            }
          }
        }
        n477 = Bundle By Name(cluster=T8 {"Enable"=[], "UCS/S"=[], "CBAL"=[], "Direction"=[], "Value"=[], "CAL"=[], "Waveform Source:"=0, "Phase Repetitions:"=0, "SYNC Sends:"=FALSE, "Delay/Pause Flag:"=FALSE, "Uncontrolled"=FALSE, "Clock Divider Enabled:"=TRUE, "Clock Divisor(n+1):"=0, "STPC"=1, "STPB+STPA"=0, "PAUSE after PHASE:"=FALSE, "Trailing Delay(n+1CLK):"=0, "Pulse Guard (n*128uS, 0=OFF)"=0, "Phase Offset:"=0, "High Voltage is:"=TRUE}, "High Voltage is:"="High Voltage is:", "Pulse Guard (n*128uS, 0=OFF)"="PG (n*128uS, 0=OFF)", "PAUSE after PHASE:"="PAUSE after PHASE:", "Trailing Delay(n+1CLK):"="Trailing Delay(n+1CLK):", "Phase Offset:"="Phase Offset:", "Clock Divider Enabled:"="Clock Divider Enabled:", "Clock Divisor(n+1):"="Clock Divisor(n+1):", "STPC"="STPC", "STPB+STPA"="STPB+STPA", "Waveform Source:"="WFM Source:", "Phase Repetitions:"="Phase Repetitions:", "SYNC Sends:"="SYNC Sends:", "Delay/Pause Flag:"="Delay/Pause Flag:", "Uncontrolled"="Uncontrolled", "Enable"=w1549, "UCS/S"=w1548, "CBAL"=w1547, "Direction"=w1546, "Value"=w1545, "CAL"=w1544) -> (w1523:T8)
        n478 = Not Equal?(x=w1523, y=w1551) -> (x != y?=w1530:bool)
        n479 = Unbundle(w1521) -> (w1526:T10)  [unwired: 22 out]
        n480 = Bundle By Name(cluster=w1522, "PHASE Changed"=w1530) -> (w1550:T1)
        n481 = Unbundle By Name(w1522) -> ("PHASE"=w1524:u8)
        n482 = Decrement(x=w1524) -> (x-1=w1519:u8)
        n483 = Replace Array Subset(array=w1526, new element=w1523, index=w1519) -> (w1525:T10)
        n484 = Bundle(cluster=w1521, w1525) -> (w1520:T11)  [unwired: 22 in]
        n485 = Index Array(array=w1528, index=w1527) -> (element=w1529:string)
      }
      frame "Clear MAIN" {
        w1745 = u8[] []  # Data
        w1746 = u16[] []  # Addresses
        w1742 = T13 {"Set RAM 1"=FALSE, "Set RAM 2"=FALSE, "RAM 1 SHAPE"=0, "RAM 2 SHAPE"=0}  # SEQ
        w1737 = T12 {"RECT 1"=255, "RECT 2"=255, "RECT 3"=255, "RECT 4"=255, "RECT 5"=255, "RECT 6"=255, "WaveDAC Ref Current"=2, "Set Basic Enables"=TRUE, "Ph/Seq/Ram Wr Ena"=TRUE, "Set WGE Bit"=TRUE, "Set All RVLD Bits"=TRUE, "Set PGOE Bit"=TRUE, "Starting Phase 0"=0, "Ending Phase 0"=1, "Starting Phase 1"=7, "Ending Phase 1"=8}  # BASE
        w1743 = T8 {"Enable"=[FALSE, FALSE, FALSE, FALSE, FALSE, FALSE, FALSE, FALSE, FALSE, FALSE, FALSE, FALSE, FALSE, FALSE, FALSE, FALSE, FALSE, FALSE, FALSE, FALSE, FALSE, FALSE, FALSE, FALSE, FALSE, FALSE], "UCS/S"=[FALSE, FALSE, FALSE, FALSE, FALSE, FALSE, FALSE, FALSE, FALSE, FALSE, FALSE, FALSE, FALSE, FALSE, FALSE, FALSE, FALSE, FALSE, FALSE, FALSE, FALSE, FALSE, FALSE, FALSE, FALSE, FALSE], "CBAL"=[FALSE, FALSE, FALSE, FALSE, FALSE, FALSE, FALSE, FALSE, FALSE, FALSE, FALSE, FALSE, FALSE, FALSE, FALSE, FALSE, FALSE, FALSE, FALSE, FALSE, FALSE, FALSE, FALSE, FALSE, FALSE, FALSE], "Direction"=[FALSE, FALSE, FALSE, FALSE, FALSE, FALSE, FALSE, FALSE, FALSE, FALSE, FALSE, FALSE, FALSE, FALSE, FALSE, FALSE, FALSE, FALSE, FALSE, FALSE, FALSE, FALSE, FALSE, FALSE, FALSE, FALSE], "Value"=[0, 0, 0, 0, 0, 0, 0, 0, 0, 0, 0, 0, 0, 0, 0, 0, 0, 0, 0, 0, 0, 0, 0, 0, 0, 0], "CAL"=[FALSE, FALSE, FALSE, FALSE, FALSE, FALSE, FALSE, FALSE, FALSE, FALSE, FALSE, FALSE, FALSE, FALSE, FALSE, FALSE, FALSE, FALSE, FALSE, FALSE, FALSE, FALSE, FALSE, FALSE, FALSE, FALSE, FALSE], "Waveform Source:"=0, "Phase Repetitions:"=0, "SYNC Sends:"=FALSE, "Delay/Pause Flag:"=FALSE, "Uncontrolled"=FALSE, "Clock Divider Enabled:"=TRUE, "Clock Divisor(n+1):"=0, "STPC"=1, "STPB+STPA"=0, "PAUSE after PHASE:"=FALSE, "Trailing Delay(n+1CLK):"=0, "Pulse Guard (n*128uS, 0=OFF)"=0, "Phase Offset:"=0, "High Voltage is:"=TRUE}  # PHASE
        n486 = Initialize Array(w1743, 24 ("dimension size")) -> (w1744:T10)
        n487 = Unbundle(w1742) -> ("Set RAM 1"=w1738:bool, "Set RAM 2"=w1739:bool, "RAM 1 SHAPE"=w1740:u16, "RAM 2 SHAPE"=w1741:u16)
        n488 = Unbundle(w1737) -> ("RECT 1"=w1721:u8, "RECT 2"=w1722:u8, "RECT 3"=w1723:u8, "RECT 4"=w1724:u8, "RECT 5"=w1725:u8, "RECT 6"=w1726:u8, "WaveDAC Ref Current"=w1727:u8, "Set Basic Enables"=w1728:bool, "Ph/Seq/Ram Wr Ena"=w1729:bool, "Set WGE Bit"=w1730:bool, "Set All RVLD Bits"=w1731:bool, "Set PGOE Bit"=w1732:bool, "Starting Phase 0"=w1733:u8, "Ending Phase 0"=w1734:u8, "Starting Phase 1"=w1735:u8, "Ending Phase 1"=w1736:u8)
        n489 = Bundle(cluster=w1748, "Set RAM 1"=w1738, "Set RAM 2"=w1739, "RAM 1 SHAPE"=w1740, "RAM 2 SHAPE"=w1741, "RECT 1"=w1721, "RECT 2"=w1722, "RECT 3"=w1723, "RECT 4"=w1724, "RECT 5"=w1725, "RECT 6"=w1726, "WaveDAC Ref Current"=w1727, "Set Basic Enables"=w1728, "Ph/Seq/Ram Wr Ena"=w1729, "Set WGE Bit"=w1730, "Set All RVLD Bits"=w1731, "Set PGOE Bit"=w1732, "Starting Phase 0"=w1733, "Ending Phase 0"=w1734, "Starting Phase 1"=w1735, "Ending Phase 1"=w1736, w1744, "Addresses"=w1746, "Data"=w1745) -> (w1747:T11)
        n490 = Index Array(array=w1751, index=w1750) -> (element=w1752:string)
      }
      frame "Write PHASE" {
        n491 = Unbundle By Name(w1757) -> ("High Voltage is:"=w1756:bool, "Waveform Source:"=w1758:u8, "Phase Repetitions:"=w1759:u8, "SYNC Sends:"=w1760:bool, "Delay/Pause Flag:"=w1761:bool, "Uncontrolled"=w1762:bool, "Clock Divider Enabled:"=w1763:bool, "Clock Divisor(n+1):"=w1764:u8, "STPC"=w1765:u8, "STPB+STPA"=w1766:u16, "PAUSE after PHASE:"=w1767:bool, "Trailing Delay(n+1CLK):"=w1768:u16, "Pulse Guard (n*128uS, 0=OFF)"=w1769:u8, "Phase Offset:"=w1770:u8, "CAL"=w1771:bool[], "Value"=w1772:u16[], "Direction"=w1773:bool[], "CBAL"=w1774:bool[], "UCS/S"=w1775:bool[], "Enable"=w1776:bool[])
        n492 = for {
          tunnel: w1776 -> [w1791] mode=indexing
          tunnel: w1775 -> [w1790] mode=indexing
          tunnel: w1774 -> [w1789] mode=indexing
          tunnel: w1773 -> [w1786] mode=indexing
          tunnel: w1772 -> [w1788] mode=indexing
          tunnel: w1771 -> [w1787] mode=indexing
          i -> [w1792]
          n493 = case shown="0, Default" w1792 {
            tunnel: w1791 -> [w1798 w1804 w1810 w1816 w1822 w1828 w1834 w1840 w1846 w1852 w1858 w1864 w1870 w1876 w1882 w1888 w1894 w1900 w1906 w1912 w1918 w1924 w1930 w1936 w1942 w1948]
            tunnel: w1790 -> [w1797 w1803 w1809 w1815 w1821 w1827 w1833 w1839 w1845 w1851 w1857 w1863 w1869 w1875 w1881 w1887 w1893 w1899 w1905 w1911 w1917 w1923 w1929 w1935 w1941 w1947]
            tunnel: w1789 -> [w1796 w1802 w1808 w1814 w1820 w1826 w1832 w1838 w1844 w1850 w1856 w1862 w1868 w1874 w1880 w1886 w1892 w1898 w1904 w1910 w1916 w1922 w1928 w1934 w1940 w1946]
            tunnel: w1788 -> [w1794 w1800 w1806 w1812 w1818 w1824 w1830 w1836 w1842 w1848 w1854 w1860 w1866 w1872 w1878 w1884 w1890 w1896 w1902 w1908 w1914 w1920 w1926 w1932 w1938 w1944]
            tunnel: w1787 -> [w1793 w1799 w1805 w1811 w1817 w1823 w1829 w1835 w1841 w1847 w1853 w1859 w1865 w1871 w1877 w1883 w1889 w1895 w1901 w1907 w1913 w1919 w1925 w1931 w1937 w1943]
            tunnel: w1786 -> [w1795 w1801 w1807 w1813 w1819 w1825 w1831 w1837 w1843 w1849 w1855 w1861 w1867 w1873 w1879 w1885 w1891 w1897 w1903 w1909 w1915 w1921 w1927 w1933 w1939 w1945]
            frame 0, Default {
              n494 = local write "Enable 1"(w1798) -> ()
              n495 = local write "UCS/S 1"(w1797) -> ()
              n496 = local write "CBAL 1"(w1796) -> ()
              n497 = local write "Direction 1"(w1795) -> ()
              n498 = local write "Value Ch 1"(w1794) -> ()
              n499 = local write "Cal 1"(w1793) -> ()
            }
            frame 1 {
              n500 = local write "Enable 2"(w1804) -> ()
              n501 = local write "UCS/S 2"(w1803) -> ()
              n502 = local write "CBAL 2"(w1802) -> ()
              n503 = local write "Direction 2"(w1801) -> ()
              n504 = local write "Value Ch 2"(w1800) -> ()
              n505 = local write "Cal 2"(w1799) -> ()
            }
            frame 2 {
              n506 = local write "Enable 3"(w1810) -> ()
              n507 = local write "UCS/S 3"(w1809) -> ()
              n508 = local write "CBAL 3"(w1808) -> ()
              n509 = local write "Direction 3"(w1807) -> ()
              n510 = local write "Value Ch 3"(w1806) -> ()
              n511 = local write "Cal 3"(w1805) -> ()
            }
            frame 3 {
              n512 = local write "Enable 4"(w1816) -> ()
              n513 = local write "UCS/S 4"(w1815) -> ()
              n514 = local write "CBAL 4"(w1814) -> ()
              n515 = local write "Direction 4"(w1813) -> ()
              n516 = local write "Value Ch 4"(w1812) -> ()
              n517 = local write "Cal 4"(w1811) -> ()
            }
            frame 4 {
              n518 = local write "Enable 5"(w1822) -> ()
              n519 = local write "UCS/S 5"(w1821) -> ()
              n520 = local write "CBAL 5"(w1820) -> ()
              n521 = local write "Direction 5"(w1819) -> ()
              n522 = local write "Value Ch 5"(w1818) -> ()
              n523 = local write "Cal 5"(w1817) -> ()
            }
            frame 5 {
              n524 = local write "Enable 6"(w1828) -> ()
              n525 = local write "UCS/S 6"(w1827) -> ()
              n526 = local write "CBAL 6"(w1826) -> ()
              n527 = local write "Direction 6"(w1825) -> ()
              n528 = local write "Value Ch 6"(w1824) -> ()
              n529 = local write "Cal 6"(w1823) -> ()
            }
            frame 6 {
              n530 = local write "Enable 7"(w1834) -> ()
              n531 = local write "UCS/S 7"(w1833) -> ()
              n532 = local write "CBAL 7"(w1832) -> ()
              n533 = local write "Direction 7"(w1831) -> ()
              n534 = local write "Value Ch 7"(w1830) -> ()
              n535 = local write "Cal 7"(w1829) -> ()
            }
            frame 7 {
              n536 = local write "Enable 8"(w1840) -> ()
              n537 = local write "UCS/S 8"(w1839) -> ()
              n538 = local write "CBAL 8"(w1838) -> ()
              n539 = local write "Direction 8"(w1837) -> ()
              n540 = local write "Value Ch 8"(w1836) -> ()
              n541 = local write "Cal 8"(w1835) -> ()
            }
            frame 8 {
              n542 = local write "Enable 9"(w1846) -> ()
              n543 = local write "UCS/S 9"(w1845) -> ()
              n544 = local write "CBAL 9"(w1844) -> ()
              n545 = local write "Direction 9"(w1843) -> ()
              n546 = local write "Value Ch 9"(w1842) -> ()
              n547 = local write "Cal 9"(w1841) -> ()
            }
            frame 9 {
              n548 = local write "Enable 10"(w1852) -> ()
              n549 = local write "UCS/S 10"(w1851) -> ()
              n550 = local write "CBAL 10"(w1850) -> ()
              n551 = local write "Direction 10"(w1849) -> ()
              n552 = local write "Value Ch 10"(w1848) -> ()
              n553 = local write "Cal 10"(w1847) -> ()
            }
            frame 10 {
              n554 = local write "Enable 11"(w1858) -> ()
              n555 = local write "UCS/S 11"(w1857) -> ()
              n556 = local write "CBAL 11"(w1856) -> ()
              n557 = local write "Direction 11"(w1855) -> ()
              n558 = local write "Value Ch 11"(w1854) -> ()
              n559 = local write "Cal 11"(w1853) -> ()
            }
            frame 11 {
              n560 = local write "Enable 12"(w1864) -> ()
              n561 = local write "UCS/S 12"(w1863) -> ()
              n562 = local write "CBAL 12"(w1862) -> ()
              n563 = local write "Direction 12"(w1861) -> ()
              n564 = local write "Value Ch 12"(w1860) -> ()
              n565 = local write "Cal 12"(w1859) -> ()
            }
            frame 12 {
              n566 = local write "Enable 13"(w1870) -> ()
              n567 = local write "UCS/S 13"(w1869) -> ()
              n568 = local write "CBAL 13"(w1868) -> ()
              n569 = local write "Direction 13"(w1867) -> ()
              n570 = local write "Value Ch 13"(w1866) -> ()
              n571 = local write "Cal 13"(w1865) -> ()
            }
            frame 13 {
              n572 = local write "Enable 14"(w1876) -> ()
              n573 = local write "UCS/S 14"(w1875) -> ()
              n574 = local write "CBAL 14"(w1874) -> ()
              n575 = local write "Direction 14"(w1873) -> ()
              n576 = local write "Value Ch 14"(w1872) -> ()
              n577 = local write "Cal 14"(w1871) -> ()
            }
            frame 14 {
              n578 = local write "Enable 15"(w1882) -> ()
              n579 = local write "UCS/S 15"(w1881) -> ()
              n580 = local write "CBAL 15"(w1880) -> ()
              n581 = local write "Direction 15"(w1879) -> ()
              n582 = local write "Value Ch 15"(w1878) -> ()
              n583 = local write "Cal 15"(w1877) -> ()
            }
            frame 15 {
              n584 = local write "Enable 16"(w1888) -> ()
              n585 = local write "UCS/S 16"(w1887) -> ()
              n586 = local write "CBAL 16"(w1886) -> ()
              n587 = local write "Direction 16"(w1885) -> ()
              n588 = local write "Value Ch 16"(w1884) -> ()
              n589 = local write "Cal 16"(w1883) -> ()
            }
            frame 16 {
              n590 = local write "Enable 17"(w1894) -> ()
              n591 = local write "UCS/S 17"(w1893) -> ()
              n592 = local write "CBAL 17"(w1892) -> ()
              n593 = local write "Direction 17"(w1891) -> ()
              n594 = local write "Value Ch 17"(w1890) -> ()
              n595 = local write "Cal 17"(w1889) -> ()
            }
            frame 17 {
              n596 = local write "Enable 18"(w1900) -> ()
              n597 = local write "UCS/S 18"(w1899) -> ()
              n598 = local write "CBAL 18"(w1898) -> ()
              n599 = local write "Direction 18"(w1897) -> ()
              n600 = local write "Value Ch 18"(w1896) -> ()
              n601 = local write "Cal 18"(w1895) -> ()
            }
            frame 18 {
              n602 = local write "Enable 19"(w1906) -> ()
              n603 = local write "UCS/S 19"(w1905) -> ()
              n604 = local write "CBAL 19"(w1904) -> ()
              n605 = local write "Direction 19"(w1903) -> ()
              n606 = local write "Value Ch 19"(w1902) -> ()
              n607 = local write "Cal 19"(w1901) -> ()
            }
            frame 19 {
              n608 = local write "Enable 20"(w1912) -> ()
              n609 = local write "UCS/S 20"(w1911) -> ()
              n610 = local write "CBAL 20"(w1910) -> ()
              n611 = local write "Direction 20"(w1909) -> ()
              n612 = local write "Value Ch 20"(w1908) -> ()
              n613 = local write "Cal 20"(w1907) -> ()
            }
            frame 20 {
              n614 = local write "Enable 21"(w1918) -> ()
              n615 = local write "UCS/S 21"(w1917) -> ()
              n616 = local write "CBAL 21"(w1916) -> ()
              n617 = local write "Direction 21"(w1915) -> ()
              n618 = local write "Value Ch 21"(w1914) -> ()
              n619 = local write "Cal 21"(w1913) -> ()
            }
            frame 21 {
              n620 = local write "Enable 22"(w1924) -> ()
              n621 = local write "UCS/S 22"(w1923) -> ()
              n622 = local write "CBAL 22"(w1922) -> ()
              n623 = local write "Direction 22"(w1921) -> ()
              n624 = local write "Value Ch 22"(w1920) -> ()
              n625 = local write "Cal 22"(w1919) -> ()
            }
            frame 22 {
              n626 = local write "Enable 23"(w1930) -> ()
              n627 = local write "UCS/S 23"(w1929) -> ()
              n628 = local write "CBAL 23"(w1928) -> ()
              n629 = local write "Direction 23"(w1927) -> ()
              n630 = local write "Value Ch 23"(w1926) -> ()
              n631 = local write "Cal 23"(w1925) -> ()
            }
            frame 23 {
              n632 = local write "Enable 24"(w1936) -> ()
              n633 = local write "UCS/S 24"(w1935) -> ()
              n634 = local write "CBAL 24"(w1934) -> ()
              n635 = local write "Direction 24"(w1933) -> ()
              n636 = local write "Value Ch 24"(w1932) -> ()
              n637 = local write "Cal 24"(w1931) -> ()
            }
            frame 24 {
              n638 = local write "Enable 25"(w1942) -> ()
              n639 = local write "UCS/S 25"(w1941) -> ()
              n640 = local write "CBAL 25"(w1940) -> ()
              n641 = local write "Direction 25"(w1939) -> ()
              n642 = local write "Value Ch 25"(w1938) -> ()
              n643 = local write "Cal 25"(w1937) -> ()
            }
            frame 25 {
              n644 = local write "Enable 26"(w1948) -> ()
              n645 = local write "UCS/S 26"(w1947) -> ()
              n646 = local write "CBAL 26"(w1946) -> ()
              n647 = local write "Direction 26"(w1945) -> ()
              n648 = local write "Value Ch 26"(w1944) -> ()
              n649 = local write "Cal 26"(w1943) -> ()
            }
          }
        }
        n650 = local write "High Voltage is:"(w1756) -> ()
        n651 = local write "Phase Repetitions:"(w1759) -> ()
        n652 = local write "SYNC Sends:"(w1760) -> ()
        n653 = local write "Delay/Pause Flag:"(w1761) -> ()
        n654 = local write "Uncontrolled"(w1762) -> ()
        n655 = local write "Clock Divider Enabled:"(w1763) -> ()
        n656 = local write "Clock Divisor(n+1):"(w1764) -> ()
        n657 = local write "STPC"(w1765) -> ()
        n658 = local write "STPB+STPA"(w1766) -> ()
        n659 = local write "PAUSE after PHASE:"(w1767) -> ()
        n660 = local write "Trailing Delay(n+1CLK):"(w1768) -> ()
        n661 = local write "Phase Offset:"(w1770) -> ()
        n662 = local write "WFM Source:"(w1758) -> ()
        n663 = local write "PG (n*128uS, 0=OFF)"(w1769) -> ()
        n664 = Index Array(array=w1780, index=w1779) -> (element=w1781:string)
      }
      frame "Write SEQ" {
        n665 = Unbundle By Name(w1957) -> ("Set RAM 1"=w1956:bool, "Set RAM 2"=w1955:bool, "RAM 1 SHAPE"=w1954:u16, "RAM 2 SHAPE"=w1953:u16)
        n666 = local write "RAM 1 SHAPE"(w1954) -> ()
        n667 = local write "RAM 2 SHAPE"(w1953) -> ()
        n668 = local write "Set RAM 1"(w1956) -> ()
        n669 = local write "Set RAM 2"(w1955) -> ()
        n670 = Index Array(array=w1951, index=w1950) -> (element=w1952:string)
      }
      frame "Read SEQ" {
        n671 = Bundle("Set RAM 1"="Set RAM 1", "Set RAM 2"="Set RAM 2", "RAM 1 SHAPE"="RAM 1 SHAPE", "RAM 2 SHAPE"="RAM 2 SHAPE") -> (w1973:T13)  [unwired: 1 in]
        n672 = Not Equal?(x=w1973, y=w1972) -> (x != y?=w1969:bool)
        n673 = Bundle(cluster=w1968, "Set RAM 1"="Set RAM 1", "Set RAM 2"="Set RAM 2", "RAM 1 SHAPE"="RAM 1 SHAPE", "RAM 2 SHAPE"="RAM 2 SHAPE") -> (w1967:T11)  [unwired: 19 in]
        n674 = Bundle By Name(cluster=w1971, "SEQ Changed"=w1969) -> (w1970:T1)
        n675 = Index Array(array=w1975, index=w1974) -> (element=w1976:string)
      }
    }
    n676 = Unbundle By Name(w20) -> ("status"=w19:bool)
    n677 = Increment(x=w11) -> (x+1=w10:i32)
    n678 = Select(t="Error", s=w19, f=w21) -> (s? t:f=w22:string)
  }
  "error out" <- w6
